vi "RDG822 User.vi"() -> ()   [LabVIEW 2021]
panel:
  in  "MenuCont":u32=1
  in  "RemoveReq?":bool=TRUE
  in  "userID":string="0001"
  out "error out":errorcluster
  in  "E:\\Study\\НИР_Маг\\FP":path=path "E:/Study/НИР_Маг/FP"
  in  "error in":errorcluster
  in  "DutyDBL":dbl=50.0 format="%.3f"
  out "DutyStr":string="50.000 %"
  in  "Noise":bool
  in  "Pulse":bool
  in  "Ramp":bool
  in  "Square":bool
  in  "Sine":bool
  in  "Slider":bool
  in  "PhaseDBL":dbl format="%.3f"
  in  "OK":bool
  out "PhaseStr":string="5.0000"
  in  "LowL":dbl=-2.5 format="%.4f"
  in  "Offset":dbl format="%.4f"
  out "Offset-LowL":string="5.0000"
  in  "Offset/LowL":bool
  in  "HighL":dbl=1.0 format="%.4f"
  in  "Ampl":dbl=5.0 format="%.4f"
  out "Ampl-HighL":string="5.0000"
  in  "Ampl/HighL":bool
  in  "Freq":dbl=1.0 format="%#_18g"
  in  "Period":dbl=1.0 format="%_8g"
  out "Freq-Period":string="1,000000000"
  in  "Freq/Period":bool
  in  "Left":bool
  in  "Right":bool
  in  "Out2":bool
  in  "Out1":bool
  out "Screen":picture
  in  "Menu":bool
  in  "Home":bool
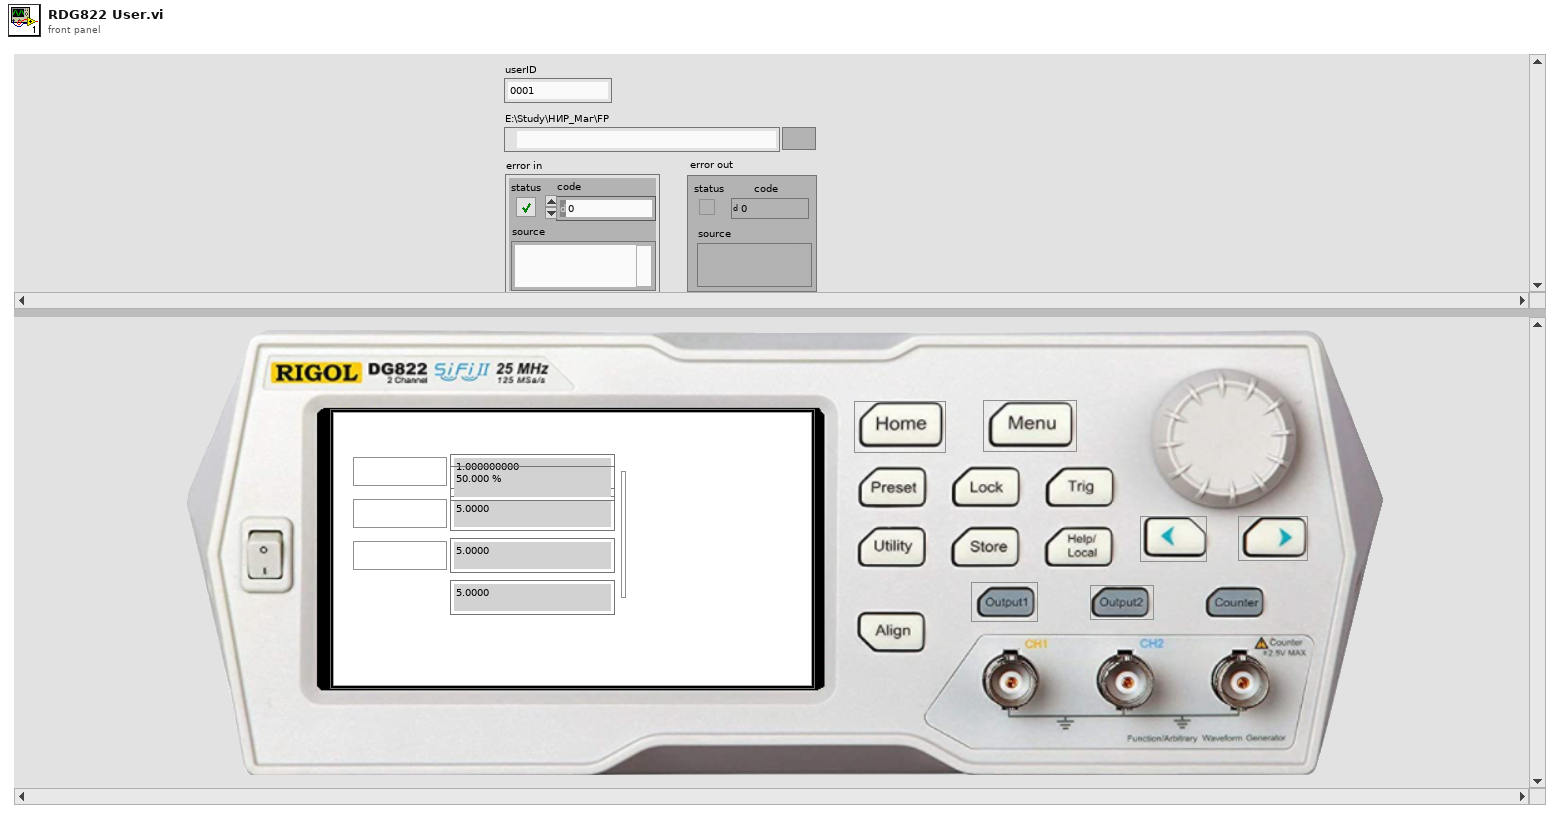
[diagram p1: front panel]
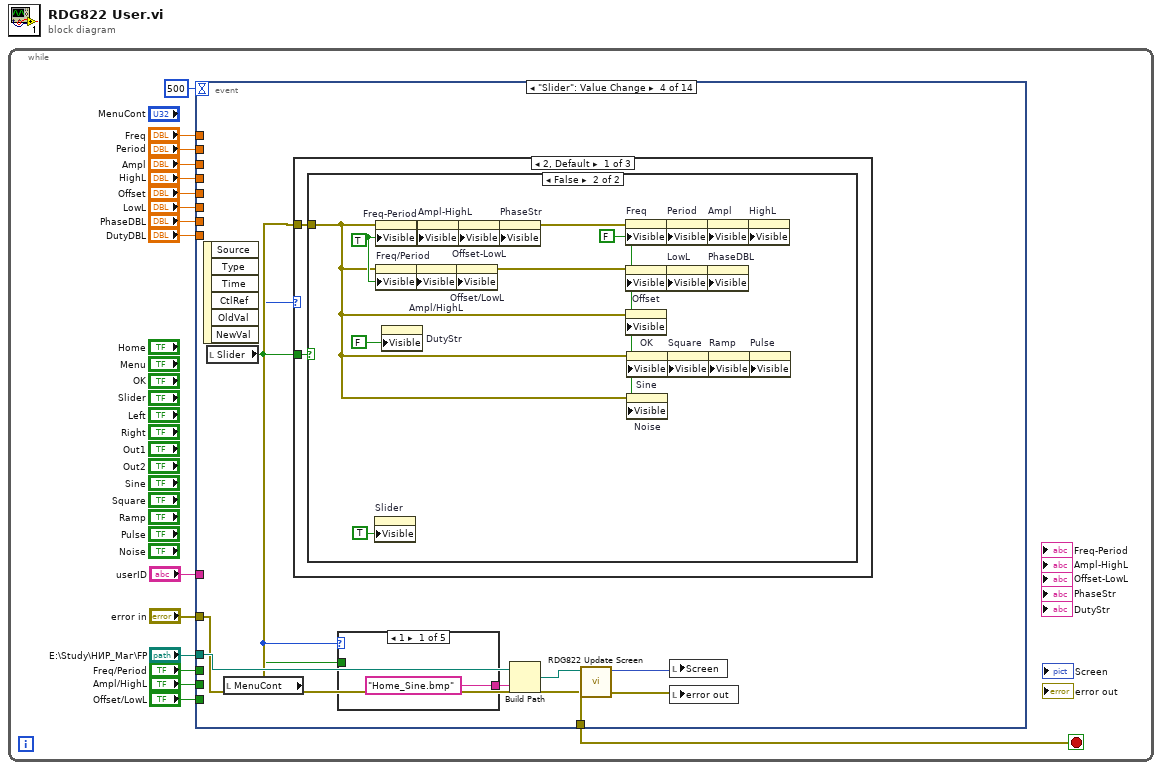
[diagram p0: block diagram]
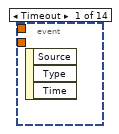
[diagram p2: hidden frame]
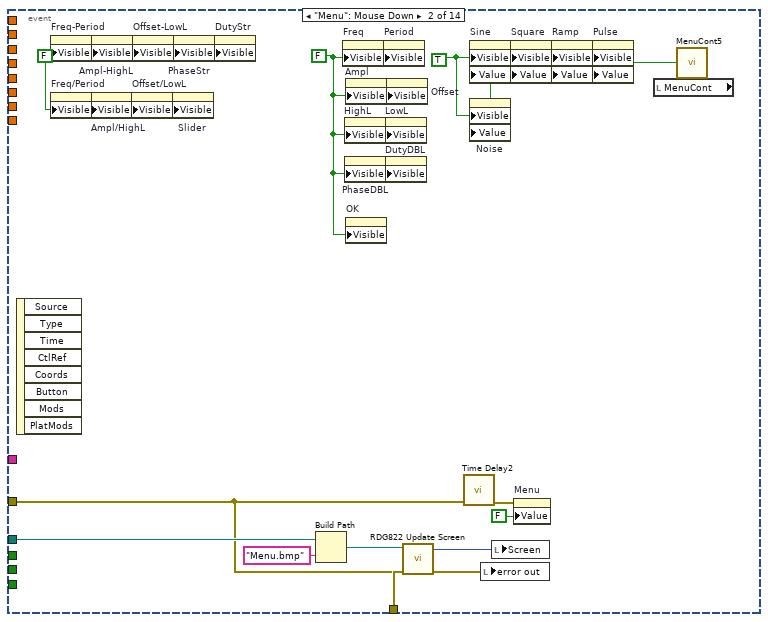
[diagram p3: hidden frame]
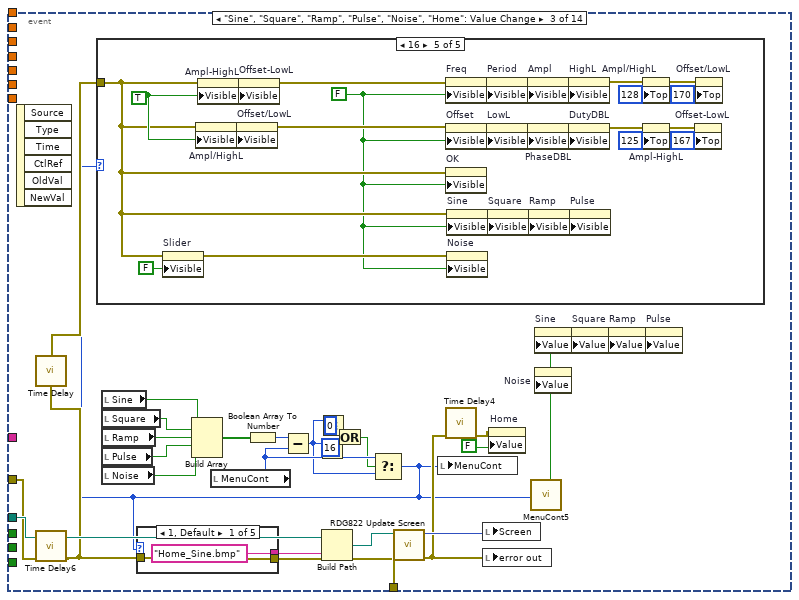
[diagram p4: hidden frame]
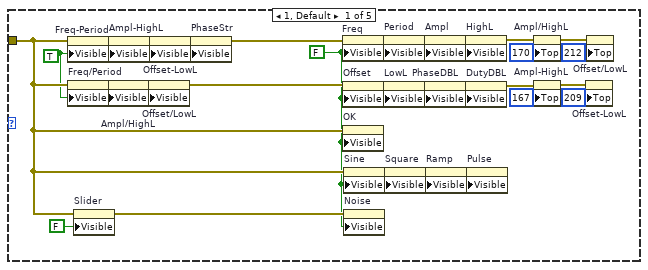
[diagram p5: hidden frame]
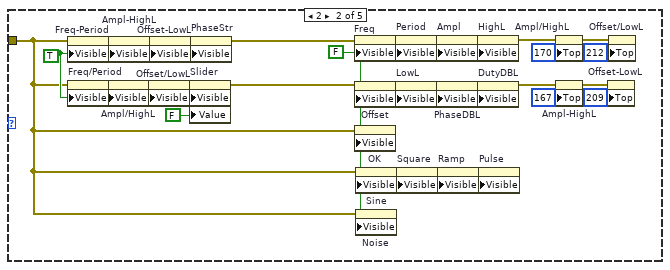
[diagram p6: hidden frame]
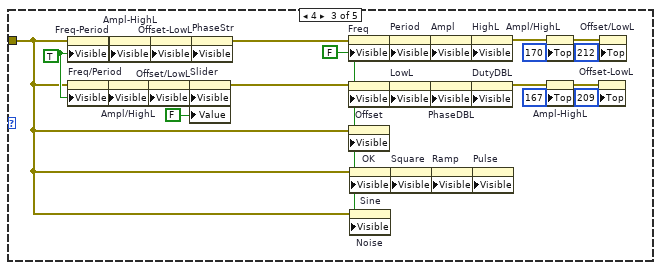
[diagram p7: hidden frame]
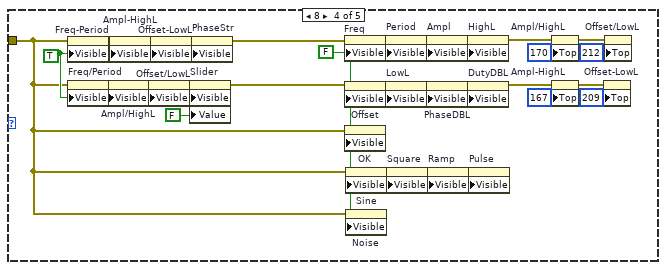
[diagram p8: hidden frame]
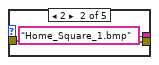
[diagram p9: hidden frame]
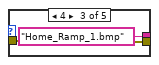
[diagram p10: hidden frame]
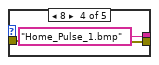
[diagram p11: hidden frame]
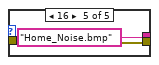
[diagram p12: hidden frame]
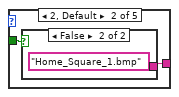
[diagram p13: hidden frame]
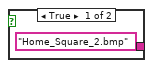
[diagram p14: hidden frame]
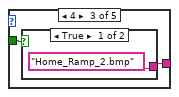
[diagram p15: hidden frame]
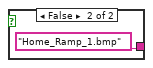
[diagram p16: hidden frame]
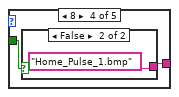
[diagram p17: hidden frame]
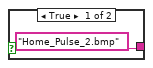
[diagram p18: hidden frame]
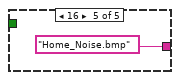
[diagram p19: hidden frame]
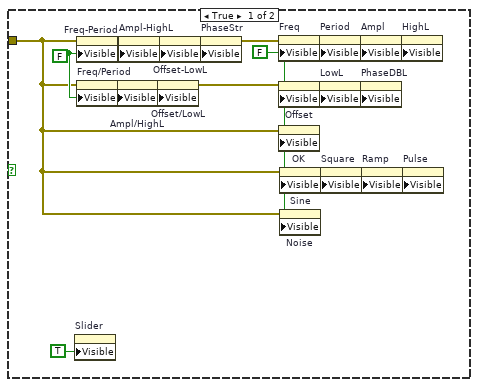
[diagram p20: hidden frame]
diagram:
  n1 = while {
    stop <- w16 stop-if-true
    n2 = event shown="[3] \"Slider\": Value Change" {
      selector: _ -> [_ _ _ _ _ _ _ _ _ _ _ _ _ _]
      dyn-events: _ -> [_ _ _ _ _ _ _ _ _ _ _ _ _ _]
      timeout: 500 -> [_ _ _ _ _ _ _ _ _ _ _ _ _ _]
      tunnel: [_ w39 w64 w229 w375 w518 w552 w587 w622 w645 _ _ w705 _] -> w16
      tunnel: "error in" -> [_ w37 w52 w228 w383 _ _ _ _ _ _ _ w723 _]
      tunnel: "E:\\Study\\НИР_Маг\\FP" -> [_ w40 w68 w230 w387 w535 w570 w605 w629 w652 _ _ w711 _]
      tunnel: "Freq/Period" -> [_ _ _ _ w390 w533 _ _ _ _ _ _ w740 _]
      tunnel: "Ampl/HighL" -> [_ _ _ _ w389 _ w565 _ _ _ _ _ w741 _]
      tunnel: "Freq" -> [_ _ _ _ _ _ _ _ _ _ _ _ w739 _]
      tunnel: "Ampl" -> [_ _ _ _ _ _ _ _ _ _ _ _ w737 _]
      tunnel: "Period" -> [_ _ _ _ _ _ _ _ _ _ _ _ w738 _]
      tunnel: "HighL" -> [_ _ _ _ _ _ _ _ _ _ _ _ w734 _]
      tunnel: "Offset/LowL" -> [_ _ _ _ w388 _ _ w593 _ _ _ _ w736 _]
      tunnel: "Offset" -> [_ _ _ _ _ _ _ _ _ _ _ _ w700 _]
      tunnel: "LowL" -> [_ _ _ _ _ _ _ _ _ _ _ _ w735 _]
      tunnel: "PhaseDBL" -> [_ _ _ _ _ _ _ _ _ _ _ _ w728 _]
      tunnel: "userID" -> [_ _ _ _ _ _ _ _ _ _ _ _ w722 _]
      tunnel: "DutyDBL" -> [_ _ _ _ _ _ _ _ _ _ _ _ w697 _]
      event Timeout {
        n3 = event-data() -> ()  [unwired: 1 in, 3 out]
      }
      event "Menu": Mouse Down {
        w25 = TRUE ("Visible")
        w18 = FALSE ("Visible")
        w17 = FALSE ("Visible")
        n4 = event-data() -> ()  [unwired: 1 in, 8 out]
        n5 = property on="Freq-Period" class="Str"("Visible"=w18) -> (error out=w36:errorcluster)  [unwired: 2 in, 1 out]
        n6 = property on="Freq/Period" class="Bool (strict)"("Visible"=w18) -> (error out=w33:errorcluster)  [unwired: 2 in, 1 out]
        n7 = property on="Ampl/HighL" class="Bool (strict)"(error in=w33, "Visible"=w18) -> (error out=w32:errorcluster)  [unwired: 1 in, 1 out]
        n8 = property on="Ampl-HighL" class="Str"(error in=w36, "Visible"=w18) -> (error out=w35:errorcluster)  [unwired: 1 in, 1 out]
        n9 = property on="Offset/LowL" class="Bool (strict)"(error in=w32, "Visible"=w18) -> (error out=w29:errorcluster)  [unwired: 1 in, 1 out]
        n10 = property on="Offset-LowL" class="Str"(error in=w35, "Visible"=w18) -> (error out=w34:errorcluster)  [unwired: 1 in, 1 out]
        n11 = property on="Slider" class="Bool (strict)"(error in=w29, "Visible"=w18) -> ()  [unwired: 1 in, 2 out]
        n12 = property on="PhaseStr" class="Str"(error in=w34, "Visible"=w18) -> ()  [unwired: 1 in, 2 out]
        n13 = property on="DutyStr" class="Str"("Visible"=w18) -> ()  [unwired: 2 in, 2 out]
        n14 = Build Path(base path=w40, name or relative path="Menu.bmp") -> (appended path=w41:path)
        n15 = property on="Freq" class="DigNum (strict)"("Visible"=w17) -> (error out=w31:errorcluster)  [unwired: 2 in, 1 out]
        n16 = property on="HighL" class="DigNum (strict)"("Visible"=w17) -> ()  [unwired: 2 in, 2 out]
        n17 = property on="PhaseDBL" class="DigNum (strict)"("Visible"=w17) -> ()  [unwired: 2 in, 2 out]
        n18 = property on="Ampl" class="DigNum (strict)"("Visible"=w17) -> (error out=w30:errorcluster)  [unwired: 2 in, 1 out]
        n19 = property on="OK" class="Bool (strict)"("Visible"=w17) -> ()  [unwired: 2 in, 2 out]
        n20 = property on="Period" class="DigNum (strict)"(error in=w31, "Visible"=w17) -> ()  [unwired: 1 in, 2 out]
        n21 = property on="LowL" class="DigNum (strict)"("Visible"=w17) -> ()  [unwired: 2 in, 2 out]
        n22 = property on="DutyDBL" class="DigNum (strict)"("Visible"=w17) -> ()  [unwired: 2 in, 2 out]
        n23 = property on="Offset" class="DigNum (strict)"(error in=w30, "Visible"=w17) -> ()  [unwired: 1 in, 2 out]
        n24 = call "RDG822 Update Screen.vi"("error in"=w37, "Path to file"=w41) -> ("error out"=w39:errorcluster, "Screen"=w38:picture)  [unwired: 8 in]
        n25 = call "Time Delay2"("error in (no error)"=w37) -> ("error out"=w44:errorcluster)  [unwired: 10 in]
        n26 = local write "error out"(w39) -> ()
        n27 = local write "Screen"(w38) -> ()
        n28 = property on="Menu" class="Bool (strict)"(error in=w44, "Value"=FALSE ("Visible")) -> ()  [unwired: 1 in, 2 out]
        n29 = local read "MenuCont"() -> (w24:u32)
        n30 = call "MenuCont5.vi"("MenuID"=w24) -> ("Sine"=w23:bool, "Square"=w22:bool, "Ramp"=w21:bool, "Pulse"=w20:bool, "Noise"=w19:bool)  [unwired: 10 in]
        n31 = property on="Sine" class="Bool (strict)"("Visible"=w25, "Value"=w23) -> (error out=w28:errorcluster)  [unwired: 2 in, 1 out]
        n32 = property on="Noise" class="Bool (strict)"("Visible"=w25, "Value"=w19) -> ()  [unwired: 2 in, 2 out]
        n33 = property on="Square" class="Bool (strict)"(error in=w28, "Visible"=w25, "Value"=w22) -> (error out=w27:errorcluster)  [unwired: 1 in, 1 out]
        n34 = property on="Ramp" class="Bool (strict)"(error in=w27, "Visible"=w25, "Value"=w21) -> (error out=w26:errorcluster)  [unwired: 1 in, 1 out]
        n35 = property on="Pulse" class="Bool (strict)"(error in=w26, "Visible"=w25, "Value"=w20) -> ()  [unwired: 1 in, 2 out]
      }
      event "Sine", "Square", "Ramp", "Pulse", "Noise", "Home": Value Change {
        n36 = event-data() -> ()  [unwired: 1 in, 6 out]
        n37 = call "Time Delay6"("error in (no error)"=w52) -> ("error out"=w49:errorcluster)  [unwired: 10 in]
        n38 = call "Time Delay"("error in (no error)"=w49) -> ("error out"=w50:errorcluster)  [unwired: 10 in]
        n39 = local read "Sine"() -> (w73:bool)
        n40 = local read "Square"() -> (w74:bool)
        n41 = local read "Ramp"() -> (w75:bool)
        n42 = local read "Pulse"() -> (w72:bool)
        n43 = local read "Noise"() -> (w71:bool)
        n44 = Build Array(w73, w74, w75, w72, w71) -> (w76:bool[])
        n45 = local read "MenuCont"() -> (w48:u32)
        n46 = Boolean Array To Number(Boolean array=w76) -> (number=w70:u32)
        n47 = Subtract(x=w70, y=w48) -> (x-y=w47:u32)
        n48 = Greater?(x=w47, y=u32 16) -> (0:w54:bool)
        n49 = Less Or Equal?(x=w47, y=u32 0) -> (x <= y?=w55:bool)
        n50 = Or(x=w55, y=w54) -> (x .or. y?=w46:bool)
        n51 = Select(t=w48, s=w46, f=w47) -> (s? t:f=w45:u32)
        n52 = case shown="16" w45 {
          tunnel: w50 -> [w90 w117 w145 w173 w200]
          frame 1, Default {
            w79 = TRUE ("Visible")
            w80 = FALSE ("Visible")
            n53 = property on="Freq-Period" class="Str"(error in=w90, "Visible"=w79) -> (error out=w106:errorcluster)  [unwired: 1 in, 1 out]
            n54 = property on="Freq/Period" class="Bool (strict)"(error in=w90, "Visible"=w79) -> (error out=w103:errorcluster)  [unwired: 1 in, 1 out]
            n55 = property on="Slider" class="Bool (strict)"(error in=w90, "Visible"=FALSE) -> (error out=w91:errorcluster)  [unwired: 1 in, 1 out]
            n56 = property on="Ampl/HighL" class="Bool (strict)"(error in=w103, "Visible"=w79) -> (error out=w102:errorcluster)  [unwired: 1 in, 1 out]
            n57 = property on="Ampl-HighL" class="Str"(error in=w106, "Visible"=w79) -> (error out=w105:errorcluster)  [unwired: 1 in, 1 out]
            n58 = property on="Offset/LowL" class="Bool (strict)"(error in=w102, "Visible"=w79) -> (error out=w92:errorcluster)  [unwired: 1 in, 1 out]
            n59 = property on="Offset-LowL" class="Str"(error in=w105, "Visible"=w79) -> (error out=w104:errorcluster)  [unwired: 1 in, 1 out]
            n60 = property on="PhaseStr" class="Str"(error in=w104, "Visible"=w79) -> (error out=w97:errorcluster)  [unwired: 1 in, 1 out]
            n61 = property on="Freq" class="DigNum (strict)"(error in=w97, "Visible"=w80) -> (error out=w96:errorcluster)  [unwired: 1 in, 1 out]
            n62 = property on="Offset" class="DigNum (strict)"(error in=w92, "Visible"=w80) -> (error out=w93:errorcluster)  [unwired: 1 in, 1 out]
            n63 = property on="OK" class="Bool (strict)"(error in=w90, "Visible"=w80) -> ()  [unwired: 1 in, 2 out]
            n64 = property on="Sine" class="Bool (strict)"(error in=w90, "Visible"=w80) -> (error out=w100:errorcluster)  [unwired: 1 in, 1 out]
            n65 = property on="Noise" class="Bool (strict)"(error in=w91, "Visible"=w80) -> ()  [unwired: 1 in, 2 out]
            n66 = property on="Period" class="DigNum (strict)"(error in=w96, "Visible"=w80) -> (error out=w95:errorcluster)  [unwired: 1 in, 1 out]
            n67 = property on="LowL" class="DigNum (strict)"(error in=w93, "Visible"=w80) -> (error out=w94:errorcluster)  [unwired: 1 in, 1 out]
            n68 = property on="Square" class="Bool (strict)"(error in=w100, "Visible"=w80) -> (error out=w99:errorcluster)  [unwired: 1 in, 1 out]
            n69 = property on="Ampl" class="DigNum (strict)"(error in=w95, "Visible"=w80) -> (error out=w101:errorcluster)  [unwired: 1 in, 1 out]
            n70 = property on="PhaseDBL" class="DigNum (strict)"(error in=w94, "Visible"=w80) -> (error out=w81:errorcluster)  [unwired: 1 in, 1 out]
            n71 = property on="Ramp" class="Bool (strict)"(error in=w99, "Visible"=w80) -> (error out=w98:errorcluster)  [unwired: 1 in, 1 out]
            n72 = property on="HighL" class="DigNum (strict)"(error in=w101, "Visible"=w80) -> (error out=w87:errorcluster)  [unwired: 1 in, 1 out]
            n73 = property on="DutyDBL" class="DigNum (strict)"("Visible"=w80) -> ()  [unwired: 2 in, 2 out]
            n74 = property on="Pulse" class="Bool (strict)"(error in=w98, "Visible"=w80) -> ()  [unwired: 1 in, 2 out]
            n75 = property on="Ampl/HighL" class="Bool (strict)"(error in=w87, "Top"=170 ("Position:Top")) -> (error out=w85:errorcluster)  [unwired: 1 in, 1 out]
            n76 = property on="Ampl-HighL" class="Str"(error in=w81, "Top"=167 ("Position:Top")) -> (error out=w82:errorcluster)  [unwired: 1 in, 1 out]
            n77 = property on="Offset-LowL" class="Str"(error in=w82, "Top"=209 ("Position:Top")) -> ()  [unwired: 1 in, 2 out]
            n78 = property on="Offset/LowL" class="Bool (strict)"(error in=w85, "Top"=212 ("Position:Top")) -> ()  [unwired: 1 in, 2 out]
          }
          frame 2 {
            w127 = TRUE ("Visible")
            w107 = FALSE ("Visible")
            n79 = property on="Freq-Period" class="Str"(error in=w117, "Visible"=w127) -> (error out=w134:errorcluster)  [unwired: 1 in, 1 out]
            n80 = property on="Freq/Period" class="Bool (strict)"(error in=w117, "Visible"=w127) -> (error out=w131:errorcluster)  [unwired: 1 in, 1 out]
            n81 = property on="Ampl/HighL" class="Bool (strict)"(error in=w131, "Visible"=w127) -> (error out=w130:errorcluster)  [unwired: 1 in, 1 out]
            n82 = property on="Ampl-HighL" class="Str"(error in=w134, "Visible"=w127) -> (error out=w133:errorcluster)  [unwired: 1 in, 1 out]
            n83 = property on="Offset/LowL" class="Bool (strict)"(error in=w130, "Visible"=w127) -> (error out=w128:errorcluster)  [unwired: 1 in, 1 out]
            n84 = property on="Offset-LowL" class="Str"(error in=w133, "Visible"=w127) -> (error out=w132:errorcluster)  [unwired: 1 in, 1 out]
            n85 = property on="Slider" class="Bool (strict)"(error in=w128, "Visible"=w127, "Value"=FALSE ("Slider")) -> (error out=w122:errorcluster)  [unwired: 1 in, 1 out]
            n86 = property on="PhaseStr" class="Str"(error in=w132, "Visible"=w127) -> (error out=w123:errorcluster)  [unwired: 1 in, 1 out]
            n87 = property on="Freq" class="DigNum (strict)"(error in=w123, "Visible"=w107) -> (error out=w121:errorcluster)  [unwired: 1 in, 1 out]
            n88 = property on="Offset" class="DigNum (strict)"(error in=w122, "Visible"=w107) -> (error out=w118:errorcluster)  [unwired: 1 in, 1 out]
            n89 = property on="OK" class="Bool (strict)"(error in=w117, "Visible"=w107) -> ()  [unwired: 1 in, 2 out]
            n90 = property on="Sine" class="Bool (strict)"(error in=w117, "Visible"=w107) -> (error out=w126:errorcluster)  [unwired: 1 in, 1 out]
            n91 = property on="Noise" class="Bool (strict)"(error in=w117, "Visible"=w107) -> ()  [unwired: 1 in, 2 out]
            n92 = property on="Period" class="DigNum (strict)"(error in=w121, "Visible"=w107) -> (error out=w120:errorcluster)  [unwired: 1 in, 1 out]
            n93 = property on="LowL" class="DigNum (strict)"(error in=w118, "Visible"=w107) -> (error out=w119:errorcluster)  [unwired: 1 in, 1 out]
            n94 = property on="Square" class="Bool (strict)"(error in=w126, "Visible"=w107) -> (error out=w125:errorcluster)  [unwired: 1 in, 1 out]
            n95 = property on="Ampl" class="DigNum (strict)"(error in=w120, "Visible"=w107) -> (error out=w129:errorcluster)  [unwired: 1 in, 1 out]
            n96 = property on="PhaseDBL" class="DigNum (strict)"(error in=w119, "Visible"=w107) -> (error out=w109:errorcluster)  [unwired: 1 in, 1 out]
            n97 = property on="Ramp" class="Bool (strict)"(error in=w125, "Visible"=w107) -> (error out=w124:errorcluster)  [unwired: 1 in, 1 out]
            n98 = property on="HighL" class="DigNum (strict)"(error in=w129, "Visible"=w107) -> (error out=w108:errorcluster)  [unwired: 1 in, 1 out]
            n99 = property on="DutyDBL" class="DigNum (strict)"("Visible"=w107) -> ()  [unwired: 2 in, 2 out]
            n100 = property on="Pulse" class="Bool (strict)"(error in=w124, "Visible"=w107) -> ()  [unwired: 1 in, 2 out]
            n101 = property on="Ampl/HighL" class="Bool (strict)"(error in=w108, "Top"=170 ("Position:Top")) -> (error out=w113:errorcluster)  [unwired: 1 in, 1 out]
            n102 = property on="Ampl-HighL" class="Str"(error in=w109, "Top"=167 ("Position:Top")) -> (error out=w110:errorcluster)  [unwired: 1 in, 1 out]
            n103 = property on="Offset-LowL" class="Str"(error in=w110, "Top"=209 ("Position:Top")) -> ()  [unwired: 1 in, 2 out]
            n104 = property on="Offset/LowL" class="Bool (strict)"(error in=w113, "Top"=212 ("Position:Top")) -> ()  [unwired: 1 in, 2 out]
          }
          frame 4 {
            w155 = TRUE ("Visible")
            w135 = FALSE ("Visible")
            n105 = property on="Freq-Period" class="Str"(error in=w145, "Visible"=w155) -> (error out=w162:errorcluster)  [unwired: 1 in, 1 out]
            n106 = property on="Freq/Period" class="Bool (strict)"(error in=w145, "Visible"=w155) -> (error out=w159:errorcluster)  [unwired: 1 in, 1 out]
            n107 = property on="Ampl/HighL" class="Bool (strict)"(error in=w159, "Visible"=w155) -> (error out=w158:errorcluster)  [unwired: 1 in, 1 out]
            n108 = property on="Ampl-HighL" class="Str"(error in=w162, "Visible"=w155) -> (error out=w161:errorcluster)  [unwired: 1 in, 1 out]
            n109 = property on="Offset/LowL" class="Bool (strict)"(error in=w158, "Visible"=w155) -> (error out=w156:errorcluster)  [unwired: 1 in, 1 out]
            n110 = property on="Offset-LowL" class="Str"(error in=w161, "Visible"=w155) -> (error out=w160:errorcluster)  [unwired: 1 in, 1 out]
            n111 = property on="Slider" class="Bool (strict)"(error in=w156, "Visible"=w155, "Value"=FALSE ("Slider")) -> (error out=w150:errorcluster)  [unwired: 1 in, 1 out]
            n112 = property on="PhaseStr" class="Str"(error in=w160, "Visible"=w155) -> (error out=w151:errorcluster)  [unwired: 1 in, 1 out]
            n113 = property on="Freq" class="DigNum (strict)"(error in=w151, "Visible"=w135) -> (error out=w149:errorcluster)  [unwired: 1 in, 1 out]
            n114 = property on="Offset" class="DigNum (strict)"(error in=w150, "Visible"=w135) -> (error out=w146:errorcluster)  [unwired: 1 in, 1 out]
            n115 = property on="OK" class="Bool (strict)"(error in=w145, "Visible"=w135) -> ()  [unwired: 1 in, 2 out]
            n116 = property on="Sine" class="Bool (strict)"(error in=w145, "Visible"=w135) -> (error out=w154:errorcluster)  [unwired: 1 in, 1 out]
            n117 = property on="Noise" class="Bool (strict)"(error in=w145, "Visible"=w135) -> ()  [unwired: 1 in, 2 out]
            n118 = property on="Period" class="DigNum (strict)"(error in=w149, "Visible"=w135) -> (error out=w148:errorcluster)  [unwired: 1 in, 1 out]
            n119 = property on="LowL" class="DigNum (strict)"(error in=w146, "Visible"=w135) -> (error out=w147:errorcluster)  [unwired: 1 in, 1 out]
            n120 = property on="Square" class="Bool (strict)"(error in=w154, "Visible"=w135) -> (error out=w153:errorcluster)  [unwired: 1 in, 1 out]
            n121 = property on="Ampl" class="DigNum (strict)"(error in=w148, "Visible"=w135) -> (error out=w157:errorcluster)  [unwired: 1 in, 1 out]
            n122 = property on="PhaseDBL" class="DigNum (strict)"(error in=w147, "Visible"=w135) -> (error out=w136:errorcluster)  [unwired: 1 in, 1 out]
            n123 = property on="Ramp" class="Bool (strict)"(error in=w153, "Visible"=w135) -> (error out=w152:errorcluster)  [unwired: 1 in, 1 out]
            n124 = property on="HighL" class="DigNum (strict)"(error in=w157, "Visible"=w135) -> (error out=w137:errorcluster)  [unwired: 1 in, 1 out]
            n125 = property on="DutyDBL" class="DigNum (strict)"("Visible"=w135) -> ()  [unwired: 2 in, 2 out]
            n126 = property on="Pulse" class="Bool (strict)"(error in=w152, "Visible"=w135) -> ()  [unwired: 1 in, 2 out]
            n127 = property on="Ampl/HighL" class="Bool (strict)"(error in=w137, "Top"=170 ("Position:Top")) -> (error out=w141:errorcluster)  [unwired: 1 in, 1 out]
            n128 = property on="Ampl-HighL" class="Str"(error in=w136, "Top"=167 ("Position:Top")) -> (error out=w138:errorcluster)  [unwired: 1 in, 1 out]
            n129 = property on="Offset-LowL" class="Str"(error in=w138, "Top"=209 ("Position:Top")) -> ()  [unwired: 1 in, 2 out]
            n130 = property on="Offset/LowL" class="Bool (strict)"(error in=w141, "Top"=212 ("Position:Top")) -> ()  [unwired: 1 in, 2 out]
          }
          frame 8 {
            w183 = TRUE ("Visible")
            w163 = FALSE ("Visible")
            n131 = property on="Freq-Period" class="Str"(error in=w173, "Visible"=w183) -> (error out=w190:errorcluster)  [unwired: 1 in, 1 out]
            n132 = property on="Freq/Period" class="Bool (strict)"(error in=w173, "Visible"=w183) -> (error out=w187:errorcluster)  [unwired: 1 in, 1 out]
            n133 = property on="Ampl/HighL" class="Bool (strict)"(error in=w187, "Visible"=w183) -> (error out=w186:errorcluster)  [unwired: 1 in, 1 out]
            n134 = property on="Ampl-HighL" class="Str"(error in=w190, "Visible"=w183) -> (error out=w189:errorcluster)  [unwired: 1 in, 1 out]
            n135 = property on="Offset/LowL" class="Bool (strict)"(error in=w186, "Visible"=w183) -> (error out=w184:errorcluster)  [unwired: 1 in, 1 out]
            n136 = property on="Offset-LowL" class="Str"(error in=w189, "Visible"=w183) -> (error out=w188:errorcluster)  [unwired: 1 in, 1 out]
            n137 = property on="Slider" class="Bool (strict)"(error in=w184, "Visible"=w183, "Value"=FALSE ("Slider")) -> (error out=w178:errorcluster)  [unwired: 1 in, 1 out]
            n138 = property on="PhaseStr" class="Str"(error in=w188, "Visible"=w183) -> (error out=w179:errorcluster)  [unwired: 1 in, 1 out]
            n139 = property on="Freq" class="DigNum (strict)"(error in=w179, "Visible"=w163) -> (error out=w177:errorcluster)  [unwired: 1 in, 1 out]
            n140 = property on="Offset" class="DigNum (strict)"(error in=w178, "Visible"=w163) -> (error out=w174:errorcluster)  [unwired: 1 in, 1 out]
            n141 = property on="OK" class="Bool (strict)"(error in=w173, "Visible"=w163) -> ()  [unwired: 1 in, 2 out]
            n142 = property on="Sine" class="Bool (strict)"(error in=w173, "Visible"=w163) -> (error out=w182:errorcluster)  [unwired: 1 in, 1 out]
            n143 = property on="Noise" class="Bool (strict)"(error in=w173, "Visible"=w163) -> ()  [unwired: 1 in, 2 out]
            n144 = property on="Period" class="DigNum (strict)"(error in=w177, "Visible"=w163) -> (error out=w176:errorcluster)  [unwired: 1 in, 1 out]
            n145 = property on="LowL" class="DigNum (strict)"(error in=w174, "Visible"=w163) -> (error out=w175:errorcluster)  [unwired: 1 in, 1 out]
            n146 = property on="Square" class="Bool (strict)"(error in=w182, "Visible"=w163) -> (error out=w181:errorcluster)  [unwired: 1 in, 1 out]
            n147 = property on="Ampl" class="DigNum (strict)"(error in=w176, "Visible"=w163) -> (error out=w185:errorcluster)  [unwired: 1 in, 1 out]
            n148 = property on="PhaseDBL" class="DigNum (strict)"(error in=w175, "Visible"=w163) -> (error out=w164:errorcluster)  [unwired: 1 in, 1 out]
            n149 = property on="Ramp" class="Bool (strict)"(error in=w181, "Visible"=w163) -> (error out=w180:errorcluster)  [unwired: 1 in, 1 out]
            n150 = property on="HighL" class="DigNum (strict)"(error in=w185, "Visible"=w163) -> (error out=w165:errorcluster)  [unwired: 1 in, 1 out]
            n151 = property on="DutyDBL" class="DigNum (strict)"("Visible"=w163) -> ()  [unwired: 2 in, 2 out]
            n152 = property on="Pulse" class="Bool (strict)"(error in=w180, "Visible"=w163) -> ()  [unwired: 1 in, 2 out]
            n153 = property on="Ampl/HighL" class="Bool (strict)"(error in=w165, "Top"=170 ("Position:Top")) -> (error out=w169:errorcluster)  [unwired: 1 in, 1 out]
            n154 = property on="Ampl-HighL" class="Str"(error in=w164, "Top"=167 ("Position:Top")) -> (error out=w166:errorcluster)  [unwired: 1 in, 1 out]
            n155 = property on="Offset-LowL" class="Str"(error in=w166, "Top"=209 ("Position:Top")) -> ()  [unwired: 1 in, 2 out]
            n156 = property on="Offset/LowL" class="Bool (strict)"(error in=w169, "Top"=212 ("Position:Top")) -> ()  [unwired: 1 in, 2 out]
          }
          frame 16 {
            w211 = TRUE ("Visible")
            w191 = FALSE ("Visible")
            n157 = property on="Slider" class="Bool (strict)"(error in=w200, "Visible"=FALSE) -> ()  [unwired: 1 in, 2 out]
            n158 = property on="Ampl/HighL" class="Bool (strict)"(error in=w200, "Visible"=w211) -> (error out=w213:errorcluster)  [unwired: 1 in, 1 out]
            n159 = property on="Ampl-HighL" class="Str"(error in=w200, "Visible"=w211) -> (error out=w214:errorcluster)  [unwired: 1 in, 1 out]
            n160 = property on="Offset/LowL" class="Bool (strict)"(error in=w213, "Visible"=w211) -> (error out=w203:errorcluster)  [unwired: 1 in, 1 out]
            n161 = property on="Offset-LowL" class="Str"(error in=w214, "Visible"=w211) -> (error out=w201:errorcluster)  [unwired: 1 in, 1 out]
            n162 = property on="Freq" class="DigNum (strict)"(error in=w201, "Visible"=w191) -> (error out=w207:errorcluster)  [unwired: 1 in, 1 out]
            n163 = property on="Offset" class="DigNum (strict)"(error in=w203, "Visible"=w191) -> (error out=w204:errorcluster)  [unwired: 1 in, 1 out]
            n164 = property on="OK" class="Bool (strict)"(error in=w200, "Visible"=w191) -> ()  [unwired: 1 in, 2 out]
            n165 = property on="Sine" class="Bool (strict)"(error in=w200, "Visible"=w191) -> (error out=w210:errorcluster)  [unwired: 1 in, 1 out]
            n166 = property on="Noise" class="Bool (strict)"(error in=w200, "Visible"=w191) -> ()  [unwired: 1 in, 2 out]
            n167 = property on="Period" class="DigNum (strict)"(error in=w207, "Visible"=w191) -> (error out=w206:errorcluster)  [unwired: 1 in, 1 out]
            n168 = property on="LowL" class="DigNum (strict)"(error in=w204, "Visible"=w191) -> (error out=w205:errorcluster)  [unwired: 1 in, 1 out]
            n169 = property on="Square" class="Bool (strict)"(error in=w210, "Visible"=w191) -> (error out=w209:errorcluster)  [unwired: 1 in, 1 out]
            n170 = property on="Ampl" class="DigNum (strict)"(error in=w206, "Visible"=w191) -> (error out=w212:errorcluster)  [unwired: 1 in, 1 out]
            n171 = property on="PhaseDBL" class="DigNum (strict)"(error in=w205, "Visible"=w191) -> (error out=w192:errorcluster)  [unwired: 1 in, 1 out]
            n172 = property on="Ramp" class="Bool (strict)"(error in=w209, "Visible"=w191) -> (error out=w208:errorcluster)  [unwired: 1 in, 1 out]
            n173 = property on="HighL" class="DigNum (strict)"(error in=w212, "Visible"=w191) -> (error out=w193:errorcluster)  [unwired: 1 in, 1 out]
            n174 = property on="DutyDBL" class="DigNum (strict)"("Visible"=w191) -> ()  [unwired: 2 in, 2 out]
            n175 = property on="Pulse" class="Bool (strict)"(error in=w208, "Visible"=w191) -> ()  [unwired: 1 in, 2 out]
            n176 = property on="Ampl/HighL" class="Bool (strict)"(error in=w193, "Top"=128 ("Position:Top")) -> (error out=w197:errorcluster)  [unwired: 1 in, 1 out]
            n177 = property on="Ampl-HighL" class="Str"(error in=w192, "Top"=125 ("Position:Top")) -> (error out=w194:errorcluster)  [unwired: 1 in, 1 out]
            n178 = property on="Offset-LowL" class="Str"(error in=w194, "Top"=167 ("Position:Top")) -> ()  [unwired: 1 in, 2 out]
            n179 = property on="Offset/LowL" class="Bool (strict)"(error in=w197, "Top"=170 ("Position:Top")) -> ()  [unwired: 1 in, 2 out]
          }
        }
        n180 = case shown="1, Default" w45 {
          tunnel: ["Home_Sine.bmp" "Home_Square_1.bmp" "Home_Ramp_1.bmp" "Home_Pulse_1.bmp" "Home_Noise.bmp"] -> w69
          tunnel: w49 -> [w215 w217 w219 w221 w223]
          tunnel: [w215 w217 w219 w221 w223] -> w51
          frame 1, Default {
          }
          frame 2 {
          }
          frame 4 {
          }
          frame 8 {
          }
          frame 16 {
          }
        }
        n181 = Build Path(base path=w68, name or relative path=w69) -> (appended path=w78:path)
        n182 = call "RDG822 Update Screen.vi"("error in"=w51, "Path to file"=w78) -> ("error out"=w64:errorcluster, "Screen"=w77:picture)  [unwired: 8 in]
        n183 = local write "MenuCont"(w45) -> ()
        n184 = call "Time Delay4"("error in (no error)"=w64) -> ("error out"=w66:errorcluster)  [unwired: 10 in]
        n185 = local write "Screen"(w77) -> ()
        n186 = local write "error out"(w64) -> ()
        n187 = property on="Home" class="Bool (strict)"(error in=w66, "Value"=FALSE ("Home")) -> ()  [unwired: 1 in, 2 out]
        n188 = call "MenuCont5.vi"("MenuID"=w45) -> ("Sine"=w60:bool, "Square"=w59:bool, "Ramp"=w58:bool, "Pulse"=w57:bool, "Noise"=w56:bool)  [unwired: 10 in]
        n189 = property on="Sine" class="Bool (strict)"("Value"=w60) -> (error out=w63:errorcluster)  [unwired: 2 in, 1 out]
        n190 = property on="Noise" class="Bool (strict)"("Value"=w56) -> ()  [unwired: 2 in, 2 out]
        n191 = property on="Square" class="Bool (strict)"(error in=w63, "Value"=w59) -> (error out=w62:errorcluster)  [unwired: 1 in, 1 out]
        n192 = property on="Ramp" class="Bool (strict)"(error in=w62, "Value"=w58) -> (error out=w61:errorcluster)  [unwired: 1 in, 1 out]
        n193 = property on="Pulse" class="Bool (strict)"(error in=w61, "Value"=w57) -> ()  [unwired: 1 in, 2 out]
      }
      event "Slider": Value Change {
        n194 = event-data() -> ()  [unwired: 1 in, 6 out]
        n195 = local read "Slider"() -> (w226:bool)
        n196 = local read "MenuCont"() -> (w227:u32)
        n197 = case shown="2, Default" w227 {
          tunnel: w228 -> [w248 w289 w329]
          tunnel: w226 -> [w247 w288 w328]
          frame 2, Default {
            n198 = case shown="False" w247 {
              tunnel: w248 -> [w251 w271]
              frame True {
                w261 = FALSE ("Visible")
                w257 = FALSE ("Visible")
                n199 = property on="Slider" class="Bool (strict)"("Visible"=TRUE) -> ()  [unwired: 2 in, 2 out]
                n200 = property on="Freq-Period" class="Str"(error in=w251, "Visible"=w261) -> (error out=w267:errorcluster)  [unwired: 1 in, 1 out]
                n201 = property on="Freq/Period" class="Bool (strict)"(error in=w251, "Visible"=w261) -> (error out=w264:errorcluster)  [unwired: 1 in, 1 out]
                n202 = property on="Ampl/HighL" class="Bool (strict)"(error in=w264, "Visible"=w261) -> (error out=w263:errorcluster)  [unwired: 1 in, 1 out]
                n203 = property on="Ampl-HighL" class="Str"(error in=w267, "Visible"=w261) -> (error out=w266:errorcluster)  [unwired: 1 in, 1 out]
                n204 = property on="Offset/LowL" class="Bool (strict)"(error in=w263, "Visible"=w261) -> (error out=w250:errorcluster)  [unwired: 1 in, 1 out]
                n205 = property on="Offset-LowL" class="Str"(error in=w266, "Visible"=w261) -> (error out=w265:errorcluster)  [unwired: 1 in, 1 out]
                n206 = property on="PhaseStr" class="Str"(error in=w265, "Visible"=w261) -> (error out=w256:errorcluster)  [unwired: 1 in, 1 out]
                n207 = property on="Freq" class="DigNum (strict)"(error in=w256, "Visible"=w257) -> (error out=w255:errorcluster)  [unwired: 1 in, 1 out]
                n208 = property on="Offset" class="DigNum (strict)"(error in=w250, "Visible"=w257) -> (error out=w252:errorcluster)  [unwired: 1 in, 1 out]
                n209 = property on="OK" class="Bool (strict)"(error in=w251, "Visible"=w257) -> ()  [unwired: 1 in, 2 out]
                n210 = property on="Sine" class="Bool (strict)"(error in=w251, "Visible"=w257) -> (error out=w260:errorcluster)  [unwired: 1 in, 1 out]
                n211 = property on="Noise" class="Bool (strict)"(error in=w251, "Visible"=w257) -> ()  [unwired: 1 in, 2 out]
                n212 = property on="Period" class="DigNum (strict)"(error in=w255, "Visible"=w257) -> (error out=w254:errorcluster)  [unwired: 1 in, 1 out]
                n213 = property on="LowL" class="DigNum (strict)"(error in=w252, "Visible"=w257) -> (error out=w253:errorcluster)  [unwired: 1 in, 1 out]
                n214 = property on="Square" class="Bool (strict)"(error in=w260, "Visible"=w257) -> (error out=w259:errorcluster)  [unwired: 1 in, 1 out]
                n215 = property on="Ampl" class="DigNum (strict)"(error in=w254, "Visible"=w257) -> (error out=w262:errorcluster)  [unwired: 1 in, 1 out]
                n216 = property on="PhaseDBL" class="DigNum (strict)"(error in=w253, "Visible"=w257) -> ()  [unwired: 1 in, 2 out]
                n217 = property on="Ramp" class="Bool (strict)"(error in=w259, "Visible"=w257) -> (error out=w258:errorcluster)  [unwired: 1 in, 1 out]
                n218 = property on="HighL" class="DigNum (strict)"(error in=w262, "Visible"=w257) -> ()  [unwired: 1 in, 2 out]
                n219 = property on="Pulse" class="Bool (strict)"(error in=w258, "Visible"=w257) -> ()  [unwired: 1 in, 2 out]
              }
              frame False {
                w281 = TRUE ("Visible")
                w277 = FALSE ("Visible")
                n220 = property on="Slider" class="Bool (strict)"("Visible"=TRUE) -> ()  [unwired: 2 in, 2 out]
                n221 = property on="Freq-Period" class="Str"(error in=w271, "Visible"=w281) -> (error out=w287:errorcluster)  [unwired: 1 in, 1 out]
                n222 = property on="Freq/Period" class="Bool (strict)"(error in=w271, "Visible"=w281) -> (error out=w284:errorcluster)  [unwired: 1 in, 1 out]
                n223 = property on="DutyStr" class="Str"("Visible"=FALSE) -> ()  [unwired: 2 in, 2 out]
                n224 = property on="Ampl/HighL" class="Bool (strict)"(error in=w284, "Visible"=w281) -> (error out=w283:errorcluster)  [unwired: 1 in, 1 out]
                n225 = property on="Ampl-HighL" class="Str"(error in=w287, "Visible"=w281) -> (error out=w286:errorcluster)  [unwired: 1 in, 1 out]
                n226 = property on="Offset/LowL" class="Bool (strict)"(error in=w283, "Visible"=w281) -> (error out=w270:errorcluster)  [unwired: 1 in, 1 out]
                n227 = property on="Offset-LowL" class="Str"(error in=w286, "Visible"=w281) -> (error out=w285:errorcluster)  [unwired: 1 in, 1 out]
                n228 = property on="PhaseStr" class="Str"(error in=w285, "Visible"=w281) -> (error out=w276:errorcluster)  [unwired: 1 in, 1 out]
                n229 = property on="Freq" class="DigNum (strict)"(error in=w276, "Visible"=w277) -> (error out=w275:errorcluster)  [unwired: 1 in, 1 out]
                n230 = property on="Offset" class="DigNum (strict)"(error in=w270, "Visible"=w277) -> (error out=w272:errorcluster)  [unwired: 1 in, 1 out]
                n231 = property on="OK" class="Bool (strict)"(error in=w271, "Visible"=w277) -> ()  [unwired: 1 in, 2 out]
                n232 = property on="Sine" class="Bool (strict)"(error in=w271, "Visible"=w277) -> (error out=w280:errorcluster)  [unwired: 1 in, 1 out]
                n233 = property on="Noise" class="Bool (strict)"(error in=w271, "Visible"=w277) -> ()  [unwired: 1 in, 2 out]
                n234 = property on="Period" class="DigNum (strict)"(error in=w275, "Visible"=w277) -> (error out=w274:errorcluster)  [unwired: 1 in, 1 out]
                n235 = property on="LowL" class="DigNum (strict)"(error in=w272, "Visible"=w277) -> (error out=w273:errorcluster)  [unwired: 1 in, 1 out]
                n236 = property on="Square" class="Bool (strict)"(error in=w280, "Visible"=w277) -> (error out=w279:errorcluster)  [unwired: 1 in, 1 out]
                n237 = property on="Ampl" class="DigNum (strict)"(error in=w274, "Visible"=w277) -> (error out=w282:errorcluster)  [unwired: 1 in, 1 out]
                n238 = property on="PhaseDBL" class="DigNum (strict)"(error in=w273, "Visible"=w277) -> ()  [unwired: 1 in, 2 out]
                n239 = property on="Ramp" class="Bool (strict)"(error in=w279, "Visible"=w277) -> (error out=w278:errorcluster)  [unwired: 1 in, 1 out]
                n240 = property on="HighL" class="DigNum (strict)"(error in=w282, "Visible"=w277) -> ()  [unwired: 1 in, 2 out]
                n241 = property on="Pulse" class="Bool (strict)"(error in=w278, "Visible"=w277) -> ()  [unwired: 1 in, 2 out]
              }
            }
          }
          frame 4 {
            n242 = case shown="False" w288 {
              tunnel: w289 -> [w292 w311]
              frame True {
                w302 = FALSE ("Visible")
                w298 = FALSE ("Visible")
                n243 = property on="Freq-Period" class="Str"(error in=w292, "Visible"=w302) -> (error out=w308:errorcluster)  [unwired: 1 in, 1 out]
                n244 = property on="Freq/Period" class="Bool (strict)"(error in=w292, "Visible"=w302) -> (error out=w305:errorcluster)  [unwired: 1 in, 1 out]
                n245 = property on="Slider" class="Bool (strict)"("Visible"=TRUE) -> ()  [unwired: 2 in, 2 out]
                n246 = property on="Ampl/HighL" class="Bool (strict)"(error in=w305, "Visible"=w302) -> (error out=w304:errorcluster)  [unwired: 1 in, 1 out]
                n247 = property on="Ampl-HighL" class="Str"(error in=w308, "Visible"=w302) -> (error out=w307:errorcluster)  [unwired: 1 in, 1 out]
                n248 = property on="Offset/LowL" class="Bool (strict)"(error in=w304, "Visible"=w302) -> (error out=w291:errorcluster)  [unwired: 1 in, 1 out]
                n249 = property on="Offset-LowL" class="Str"(error in=w307, "Visible"=w302) -> (error out=w306:errorcluster)  [unwired: 1 in, 1 out]
                n250 = property on="PhaseStr" class="Str"(error in=w306, "Visible"=w302) -> (error out=w297:errorcluster)  [unwired: 1 in, 1 out]
                n251 = property on="Freq" class="DigNum (strict)"(error in=w297, "Visible"=w298) -> (error out=w296:errorcluster)  [unwired: 1 in, 1 out]
                n252 = property on="Offset" class="DigNum (strict)"(error in=w291, "Visible"=w298) -> (error out=w293:errorcluster)  [unwired: 1 in, 1 out]
                n253 = property on="OK" class="Bool (strict)"(error in=w292, "Visible"=w298) -> ()  [unwired: 1 in, 2 out]
                n254 = property on="Sine" class="Bool (strict)"(error in=w292, "Visible"=w298) -> (error out=w301:errorcluster)  [unwired: 1 in, 1 out]
                n255 = property on="Noise" class="Bool (strict)"(error in=w292, "Visible"=w298) -> ()  [unwired: 1 in, 2 out]
                n256 = property on="Period" class="DigNum (strict)"(error in=w296, "Visible"=w298) -> (error out=w295:errorcluster)  [unwired: 1 in, 1 out]
                n257 = property on="LowL" class="DigNum (strict)"(error in=w293, "Visible"=w298) -> (error out=w294:errorcluster)  [unwired: 1 in, 1 out]
                n258 = property on="Square" class="Bool (strict)"(error in=w301, "Visible"=w298) -> (error out=w300:errorcluster)  [unwired: 1 in, 1 out]
                n259 = property on="Ampl" class="DigNum (strict)"(error in=w295, "Visible"=w298) -> (error out=w303:errorcluster)  [unwired: 1 in, 1 out]
                n260 = property on="PhaseDBL" class="DigNum (strict)"(error in=w294, "Visible"=w298) -> ()  [unwired: 1 in, 2 out]
                n261 = property on="Ramp" class="Bool (strict)"(error in=w300, "Visible"=w298) -> (error out=w299:errorcluster)  [unwired: 1 in, 1 out]
                n262 = property on="HighL" class="DigNum (strict)"(error in=w303, "Visible"=w298) -> ()  [unwired: 1 in, 2 out]
                n263 = property on="Pulse" class="Bool (strict)"(error in=w299, "Visible"=w298) -> ()  [unwired: 1 in, 2 out]
              }
              frame False {
                w321 = TRUE ("Visible")
                w317 = FALSE ("Visible")
                n264 = property on="Freq-Period" class="Str"(error in=w311, "Visible"=w321) -> (error out=w327:errorcluster)  [unwired: 1 in, 1 out]
                n265 = property on="Freq/Period" class="Bool (strict)"(error in=w311, "Visible"=w321) -> (error out=w324:errorcluster)  [unwired: 1 in, 1 out]
                n266 = property on="Slider" class="Bool (strict)"("Visible"=TRUE) -> ()  [unwired: 2 in, 2 out]
                n267 = property on="Ampl/HighL" class="Bool (strict)"(error in=w324, "Visible"=w321) -> (error out=w323:errorcluster)  [unwired: 1 in, 1 out]
                n268 = property on="Ampl-HighL" class="Str"(error in=w327, "Visible"=w321) -> (error out=w326:errorcluster)  [unwired: 1 in, 1 out]
                n269 = property on="Offset/LowL" class="Bool (strict)"(error in=w323, "Visible"=w321) -> (error out=w310:errorcluster)  [unwired: 1 in, 1 out]
                n270 = property on="Offset-LowL" class="Str"(error in=w326, "Visible"=w321) -> (error out=w325:errorcluster)  [unwired: 1 in, 1 out]
                n271 = property on="PhaseStr" class="Str"(error in=w325, "Visible"=w321) -> (error out=w316:errorcluster)  [unwired: 1 in, 1 out]
                n272 = property on="Freq" class="DigNum (strict)"(error in=w316, "Visible"=w317) -> (error out=w315:errorcluster)  [unwired: 1 in, 1 out]
                n273 = property on="Offset" class="DigNum (strict)"(error in=w310, "Visible"=w317) -> (error out=w312:errorcluster)  [unwired: 1 in, 1 out]
                n274 = property on="OK" class="Bool (strict)"(error in=w311, "Visible"=w317) -> ()  [unwired: 1 in, 2 out]
                n275 = property on="Sine" class="Bool (strict)"(error in=w311, "Visible"=w317) -> (error out=w320:errorcluster)  [unwired: 1 in, 1 out]
                n276 = property on="Noise" class="Bool (strict)"(error in=w311, "Visible"=w317) -> ()  [unwired: 1 in, 2 out]
                n277 = property on="Period" class="DigNum (strict)"(error in=w315, "Visible"=w317) -> (error out=w314:errorcluster)  [unwired: 1 in, 1 out]
                n278 = property on="LowL" class="DigNum (strict)"(error in=w312, "Visible"=w317) -> (error out=w313:errorcluster)  [unwired: 1 in, 1 out]
                n279 = property on="Square" class="Bool (strict)"(error in=w320, "Visible"=w317) -> (error out=w319:errorcluster)  [unwired: 1 in, 1 out]
                n280 = property on="Ampl" class="DigNum (strict)"(error in=w314, "Visible"=w317) -> (error out=w322:errorcluster)  [unwired: 1 in, 1 out]
                n281 = property on="PhaseDBL" class="DigNum (strict)"(error in=w313, "Visible"=w317) -> ()  [unwired: 1 in, 2 out]
                n282 = property on="Ramp" class="Bool (strict)"(error in=w319, "Visible"=w317) -> (error out=w318:errorcluster)  [unwired: 1 in, 1 out]
                n283 = property on="HighL" class="DigNum (strict)"(error in=w322, "Visible"=w317) -> ()  [unwired: 1 in, 2 out]
                n284 = property on="Pulse" class="Bool (strict)"(error in=w318, "Visible"=w317) -> ()  [unwired: 1 in, 2 out]
              }
            }
          }
          frame 8 {
            n285 = case shown="True" w328 {
              tunnel: w329 -> [w332 w351]
              frame True {
                w342 = FALSE ("Visible")
                w338 = FALSE ("Visible")
                n286 = property on="Freq-Period" class="Str"(error in=w332, "Visible"=w342) -> (error out=w348:errorcluster)  [unwired: 1 in, 1 out]
                n287 = property on="Freq/Period" class="Bool (strict)"(error in=w332, "Visible"=w342) -> (error out=w345:errorcluster)  [unwired: 1 in, 1 out]
                n288 = property on="Slider" class="Bool (strict)"("Visible"=TRUE) -> ()  [unwired: 2 in, 2 out]
                n289 = property on="Ampl/HighL" class="Bool (strict)"(error in=w345, "Visible"=w342) -> (error out=w344:errorcluster)  [unwired: 1 in, 1 out]
                n290 = property on="Ampl-HighL" class="Str"(error in=w348, "Visible"=w342) -> (error out=w347:errorcluster)  [unwired: 1 in, 1 out]
                n291 = property on="Offset/LowL" class="Bool (strict)"(error in=w344, "Visible"=w342) -> (error out=w331:errorcluster)  [unwired: 1 in, 1 out]
                n292 = property on="Offset-LowL" class="Str"(error in=w347, "Visible"=w342) -> (error out=w346:errorcluster)  [unwired: 1 in, 1 out]
                n293 = property on="PhaseStr" class="Str"(error in=w346, "Visible"=w342) -> (error out=w337:errorcluster)  [unwired: 1 in, 1 out]
                n294 = property on="Freq" class="DigNum (strict)"(error in=w337, "Visible"=w338) -> (error out=w336:errorcluster)  [unwired: 1 in, 1 out]
                n295 = property on="Offset" class="DigNum (strict)"(error in=w331, "Visible"=w338) -> (error out=w333:errorcluster)  [unwired: 1 in, 1 out]
                n296 = property on="OK" class="Bool (strict)"(error in=w332, "Visible"=w338) -> ()  [unwired: 1 in, 2 out]
                n297 = property on="Sine" class="Bool (strict)"(error in=w332, "Visible"=w338) -> (error out=w341:errorcluster)  [unwired: 1 in, 1 out]
                n298 = property on="Noise" class="Bool (strict)"(error in=w332, "Visible"=w338) -> ()  [unwired: 1 in, 2 out]
                n299 = property on="Period" class="DigNum (strict)"(error in=w336, "Visible"=w338) -> (error out=w335:errorcluster)  [unwired: 1 in, 1 out]
                n300 = property on="LowL" class="DigNum (strict)"(error in=w333, "Visible"=w338) -> (error out=w334:errorcluster)  [unwired: 1 in, 1 out]
                n301 = property on="Square" class="Bool (strict)"(error in=w341, "Visible"=w338) -> (error out=w340:errorcluster)  [unwired: 1 in, 1 out]
                n302 = property on="Ampl" class="DigNum (strict)"(error in=w335, "Visible"=w338) -> (error out=w343:errorcluster)  [unwired: 1 in, 1 out]
                n303 = property on="PhaseDBL" class="DigNum (strict)"(error in=w334, "Visible"=w338) -> ()  [unwired: 1 in, 2 out]
                n304 = property on="Ramp" class="Bool (strict)"(error in=w340, "Visible"=w338) -> (error out=w339:errorcluster)  [unwired: 1 in, 1 out]
                n305 = property on="HighL" class="DigNum (strict)"(error in=w343, "Visible"=w338) -> ()  [unwired: 1 in, 2 out]
                n306 = property on="Pulse" class="Bool (strict)"(error in=w339, "Visible"=w338) -> ()  [unwired: 1 in, 2 out]
              }
              frame False {
                w361 = TRUE ("Visible")
                w357 = FALSE ("Visible")
                n307 = property on="Freq-Period" class="Str"(error in=w351, "Visible"=w361) -> (error out=w367:errorcluster)  [unwired: 1 in, 1 out]
                n308 = property on="Freq/Period" class="Bool (strict)"(error in=w351, "Visible"=w361) -> (error out=w364:errorcluster)  [unwired: 1 in, 1 out]
                n309 = property on="Slider" class="Bool (strict)"("Visible"=TRUE) -> ()  [unwired: 2 in, 2 out]
                n310 = property on="Ampl/HighL" class="Bool (strict)"(error in=w364, "Visible"=w361) -> (error out=w363:errorcluster)  [unwired: 1 in, 1 out]
                n311 = property on="Ampl-HighL" class="Str"(error in=w367, "Visible"=w361) -> (error out=w366:errorcluster)  [unwired: 1 in, 1 out]
                n312 = property on="Offset/LowL" class="Bool (strict)"(error in=w363, "Visible"=w361) -> (error out=w350:errorcluster)  [unwired: 1 in, 1 out]
                n313 = property on="Offset-LowL" class="Str"(error in=w366, "Visible"=w361) -> (error out=w365:errorcluster)  [unwired: 1 in, 1 out]
                n314 = property on="PhaseStr" class="Str"(error in=w365, "Visible"=w361) -> (error out=w356:errorcluster)  [unwired: 1 in, 1 out]
                n315 = property on="Freq" class="DigNum (strict)"(error in=w356, "Visible"=w357) -> (error out=w355:errorcluster)  [unwired: 1 in, 1 out]
                n316 = property on="Offset" class="DigNum (strict)"(error in=w350, "Visible"=w357) -> (error out=w352:errorcluster)  [unwired: 1 in, 1 out]
                n317 = property on="OK" class="Bool (strict)"(error in=w351, "Visible"=w357) -> ()  [unwired: 1 in, 2 out]
                n318 = property on="Sine" class="Bool (strict)"(error in=w351, "Visible"=w357) -> (error out=w360:errorcluster)  [unwired: 1 in, 1 out]
                n319 = property on="Noise" class="Bool (strict)"(error in=w351, "Visible"=w357) -> ()  [unwired: 1 in, 2 out]
                n320 = property on="Period" class="DigNum (strict)"(error in=w355, "Visible"=w357) -> (error out=w354:errorcluster)  [unwired: 1 in, 1 out]
                n321 = property on="LowL" class="DigNum (strict)"(error in=w352, "Visible"=w357) -> (error out=w353:errorcluster)  [unwired: 1 in, 1 out]
                n322 = property on="Square" class="Bool (strict)"(error in=w360, "Visible"=w357) -> (error out=w359:errorcluster)  [unwired: 1 in, 1 out]
                n323 = property on="Ampl" class="DigNum (strict)"(error in=w354, "Visible"=w357) -> (error out=w362:errorcluster)  [unwired: 1 in, 1 out]
                n324 = property on="PhaseDBL" class="DigNum (strict)"(error in=w353, "Visible"=w357) -> ()  [unwired: 1 in, 2 out]
                n325 = property on="Ramp" class="Bool (strict)"(error in=w359, "Visible"=w357) -> (error out=w358:errorcluster)  [unwired: 1 in, 1 out]
                n326 = property on="HighL" class="DigNum (strict)"(error in=w362, "Visible"=w357) -> ()  [unwired: 1 in, 2 out]
                n327 = property on="Pulse" class="Bool (strict)"(error in=w358, "Visible"=w357) -> ()  [unwired: 1 in, 2 out]
              }
            }
          }
        }
        n328 = case shown="1" w227 {
          tunnel: ["Home_Sine.bmp" w235 w239 w243 "Home_Noise.bmp"] -> w225
          tunnel: w226 -> [_ w234 w238 w242 _]
          frame 1 {
          }
          frame 2, Default {
            n329 = case shown="False" w234 {
              tunnel: ["Home_Square_2.bmp" "Home_Square_1.bmp"] -> w235
              frame True {
              }
              frame False {
              }
            }
          }
          frame 4 {
            n330 = case shown="True" w238 {
              tunnel: ["Home_Ramp_2.bmp" "Home_Ramp_1.bmp"] -> w239
              frame True {
              }
              frame False {
              }
            }
          }
          frame 8 {
            n331 = case shown="False" w242 {
              tunnel: ["Home_Pulse_2.bmp" "Home_Pulse_1.bmp"] -> w243
              frame True {
              }
              frame False {
              }
            }
          }
          frame 16 {
          }
        }
        n332 = Build Path(base path=w230, name or relative path=w225) -> (appended path=w232:path)
        n333 = call "RDG822 Update Screen.vi"("error in"=w228, "Path to file"=w232) -> ("error out"=w229:errorcluster, "Screen"=w231:picture)  [unwired: 8 in]
        n334 = local write "Screen"(w231) -> ()
        n335 = local write "error out"(w229) -> ()
      }
      event "OK": Mouse Down {
        w369 = TRUE ("Visible")
        w368 = FALSE ("Visible")
        # "Добавить слайдер/меню кейсы"
        # "Сделать пересчет"
        n336 = event-data() -> ()  [unwired: 1 in, 8 out]
        n337 = local read "MenuCont"() -> (w380:u32)
        n338 = local read "Slider"() -> (w382:bool)
        n339 = call "Time Delay9"("error in (no error)"=w383) -> ("error out"=w378:errorcluster)  [unwired: 10 in]
        n340 = case shown="1" w380 {
          tunnel: ["Home_Sine.bmp" w410 w417 w424 "Home_Noise.bmp"] -> w381
          tunnel: w382 -> [_ w409 w416 w423 _]
          tunnel: w378 -> [w403 w407 w414 w421 w428]
          tunnel: [w402 w406 w413 w420 w427] -> w377
          frame 1 {
            n341 = property on="Slider" class="Bool (strict)"(error in=w403, "Visible"=FALSE) -> (error out=w402:errorcluster)  [unwired: 1 in, 1 out]
          }
          frame 2, Default {
            n342 = case shown="False" w409 {
              tunnel: ["Home_Square_2.bmp" "Home_Square_1.bmp"] -> w410
              frame True {
              }
              frame False {
              }
            }
            n343 = property on="Slider" class="Bool (strict)"(error in=w407, "Visible"=TRUE) -> (error out=w406:errorcluster)  [unwired: 1 in, 1 out]
          }
          frame 4 {
            n344 = case shown="True" w416 {
              tunnel: ["Home_Ramp_2.bmp" "Home_Ramp_1.bmp"] -> w417
              frame True {
              }
              frame False {
              }
            }
            n345 = property on="Slider" class="Bool (strict)"(error in=w414, "Visible"=TRUE) -> (error out=w413:errorcluster)  [unwired: 1 in, 1 out]
          }
          frame 8 {
            n346 = case shown="False" w423 {
              tunnel: ["Home_Pulse_2.bmp" "Home_Pulse_1.bmp"] -> w424
              frame True {
              }
              frame False {
              }
            }
            n347 = property on="Slider" class="Bool (strict)"(error in=w421, "Visible"=TRUE) -> (error out=w420:errorcluster)  [unwired: 1 in, 1 out]
          }
          frame 16 {
            n348 = property on="Slider" class="Bool (strict)"(error in=w428, "Visible"=FALSE) -> (error out=w427:errorcluster)  [unwired: 1 in, 1 out]
          }
        }
        n349 = Build Path(base path=w387, name or relative path=w381) -> (appended path=w386:path)
        n350 = property on="DutyStr" class="Str"("Visible"=w369) -> ()  [unwired: 2 in, 2 out]
        n351 = call "RDG822 Update Screen.vi"("error in"=w377, "Path to file"=w386) -> ("error out"=w375:errorcluster, "Screen"=w385:picture)  [unwired: 8 in]
        n352 = property on="Freq-Period" class="Str"(error in=w375, "Visible"=w369) -> (error out=w400:errorcluster)  [unwired: 1 in, 1 out]
        n353 = property on="Ampl-HighL" class="Str"(error in=w400, "Visible"=w369) -> (error out=w399:errorcluster)  [unwired: 1 in, 1 out]
        n354 = property on="Offset-LowL" class="Str"(error in=w399, "Visible"=w369) -> (error out=w398:errorcluster)  [unwired: 1 in, 1 out]
        n355 = property on="PhaseStr" class="Str"(error in=w398, "Visible"=w369) -> (error out=w397:errorcluster)  [unwired: 1 in, 1 out]
        n356 = property on="Freq/Period" class="Bool (strict)"(error in=w397, "Visible"=w369) -> (error out=w396:errorcluster)  [unwired: 1 in, 1 out]
        n357 = property on="Ampl/HighL" class="Bool (strict)"(error in=w396, "Visible"=w369) -> (error out=w395:errorcluster)  [unwired: 1 in, 1 out]
        n358 = property on="Offset/LowL" class="Bool (strict)"(error in=w395, "Visible"=w369) -> (error out=w379:errorcluster)  [unwired: 1 in, 1 out]
        n359 = stacked-sequence {
          tunnel: [_ _ w462 _ _] -> w372
          tunnel: [_ w449 _ _ _] -> w373
          tunnel: [w432 _ _ _ _] -> w374
          tunnel: w390 -> [w431 _ _ _ _]
          tunnel: w389 -> [_ w448 _ _ _]
          tunnel: w388 -> [_ _ w461 _ _]
          tunnel: [_ w447 _ _ _] -> w376
          tunnel: w375 -> [_ w447 _ _ _]
          tunnel: [_ _ _ w469 _] -> w371
          tunnel: [_ _ _ _ w492] -> w370
          frame #0 {
            n360 = case shown="False" w431 {
              tunnel: [w434 w441] -> w432
              frame False {
                n361 = local read "Freq"() -> (w437:dbl)
                n362 = Divide(x=1000.0, y=w437) -> (x/y=w436:dbl)
                n363 = Number To Fractional String(number=w437, precision (6)=i16 9) -> (F-format string=w433:string)  [unwired: 2 in]
                n364 = local write "Period"(w436) -> ()
                n365 = Concatenate Strings(w433, " Hz" ("string")) -> (w434:string)
              }
              frame True {
                n366 = local read "Period"() -> (w444:dbl)
                n367 = Divide(x=1000.0, y=w444) -> (x/y=w443:dbl)
                n368 = Number To Fractional String(number=w444, precision (6)=i16 7) -> (F-format string=w440:string)  [unwired: 2 in]
                n369 = local write "Freq"(w443) -> ()
                n370 = Concatenate Strings(w440, " ms" ("string")) -> (w441:string)
              }
            }
          }
          frame #1 {
            n371 = case shown="False" w448 {
              tunnel: [w455 w458] -> w449
              frame False {
                # "Must vary"
                n372 = local read "Ampl"() -> (w454:dbl)
                n373 = In Range and Coerce(upper limit=20.0, x=w454, lower limit=0.002 ("t")) -> (coerced(x)=w451:dbl, In Range?=w450:bool)
                n374 = case shown="False" w450 {
                  frame False {
                    n375 = One Button Dialog(message="Amplitude can`t be less than 2 mA\nor more  than 20 A!") -> ()  [unwired: 1 in, 1 out]
                  }
                  frame True {
                  }
                }
                n376 = Number To Fractional String(number=w451, precision (6)=i16 4) -> (F-format string=w455:string)  [unwired: 2 in]
              }
              frame True {
                n377 = local read "HighL"() -> (w459:dbl)
                n378 = Number To Fractional String(number=w459, precision (6)=i16 4) -> (F-format string=w458:string)  [unwired: 2 in]
              }
            }
          }
          frame #2 {
            n379 = case shown="False" w461 {
              tunnel: [w464 w468] -> w462
              frame False {
                # "Must vary"
                n380 = local read "Offset"() -> (w465:dbl)
                n381 = Number To Fractional String(number=w465, precision (6)=i16 4) -> (F-format string=w464:string)  [unwired: 2 in]
              }
              frame True {
                n382 = local read "LowL"() -> (w466:dbl)
                n383 = Number To Fractional String(number=w466, precision (6)=i16 4) -> (F-format string=w468:string)  [unwired: 2 in]
              }
            }
          }
          frame #3 {
            n384 = local read "PhaseDBL"() -> (w473:dbl)
            n385 = while {
              shift-right: [w475] -> w472
              shift-left: w473 -> [w477]
              stop <- w476 stop-if-true
              w478 = 360.0001 ("upper limit")
              n386 = In Range and Coerce(upper limit=w478, x=w477, lower limit=0.0) -> (In Range?=w476:bool)  [unwired: 1 out]
              n387 = case shown="False" w476 {
                tunnel: w478 -> [w483 _]
                tunnel: w477 -> [w481 w490]
                tunnel: [w480 w490] -> w475
                frame False {
                  n388 = Greater?(x=w481, y=w483) -> (0:w482:bool)
                  n389 = case shown="True" w482 {
                    tunnel: w481 -> [w485 w487]
                    tunnel: [w484 w488] -> w480
                    frame False {
                      n390 = Add(x=w485, y=360.0) -> (x+y=w484:dbl)
                    }
                    frame True {
                      n391 = Subtract(x=w487, y=360.0) -> (x-y=w488:dbl)
                    }
                  }
                }
                frame True {
                }
              }
            }
            n392 = Number To Fractional String(number=w472, precision (6)=i16 3) -> (F-format string=w470:string)  [unwired: 2 in]
            n393 = Concatenate Strings(w470, " °" ("string")) -> (w469:string)
          }
          frame #4 {
            n394 = local read "DutyDBL"() -> (w495:dbl)
            n395 = while {
              shift-right: [w497] -> w494
              shift-left: w495 -> [w499]
              stop <- w498 stop-if-true
              w500 = 100.0001 ("upper limit")
              n396 = In Range and Coerce(upper limit=w500, x=w499, lower limit=0.0) -> (In Range?=w498:bool)  [unwired: 1 out]
              n397 = case shown="False" w498 {
                tunnel: w500 -> [w505 _]
                tunnel: w499 -> [w503 w512]
                tunnel: [w502 w512] -> w497
                frame False {
                  n398 = Greater?(x=w503, y=w505) -> (0:w504:bool)
                  n399 = case shown="False" w504 {
                    tunnel: w503 -> [w507 w509]
                    tunnel: [w506 w510] -> w502
                    frame False {
                      n400 = Add(x=w507, y=100.0) -> (x+y=w506:dbl)
                    }
                    frame True {
                      n401 = Subtract(x=w509, y=100.0) -> (x-y=w510:dbl)
                    }
                  }
                }
                frame True {
                }
              }
            }
            n402 = Number To Fractional String(number=w494, precision (6)=i16 3) -> (F-format string=w491:string)  [unwired: 2 in]
            n403 = Concatenate Strings(w491, " %" ("string")) -> (w492:string)
          }
        }
        n404 = property on="Offset" class="DigNum (strict)"("Visible"=w368) -> (error out=w391:errorcluster)  [unwired: 2 in, 1 out]
        n405 = property on="PhaseDBL" class="DigNum (strict)"("Visible"=w368) -> ()  [unwired: 2 in, 2 out]
        n406 = property on="Freq" class="DigNum (strict)"(error in=w379, "Visible"=w368) -> (error out=w394:errorcluster)  [unwired: 1 in, 1 out]
        n407 = property on="OK" class="Bool (strict)"("Visible"=w368) -> (error out=w384:errorcluster)  [unwired: 2 in, 1 out]
        n408 = property on="LowL" class="DigNum (strict)"(error in=w391, "Visible"=w368) -> ()  [unwired: 1 in, 2 out]
        n409 = property on="DutyDBL" class="DigNum (strict)"("Visible"=w368) -> ()  [unwired: 2 in, 2 out]
        n410 = property on="Period" class="DigNum (strict)"(error in=w394, "Visible"=w368) -> (error out=w393:errorcluster)  [unwired: 1 in, 1 out]
        n411 = property on="Ampl" class="DigNum (strict)"(error in=w393, "Visible"=w368) -> (error out=w392:errorcluster)  [unwired: 1 in, 1 out]
        n412 = property on="HighL" class="DigNum (strict)"(error in=w392, "Visible"=w368) -> ()  [unwired: 1 in, 2 out]
        n413 = call "Time Delay3"("error in (no error)"=w384) -> ("error out"=w401:errorcluster)  [unwired: 10 in]
        n414 = property on="OK" class="Bool (strict)"(error in=w401, "Value"=w368) -> ()  [unwired: 1 in, 2 out]
        n415 = local write "Freq-Period"(w374) -> ()
        n416 = local write "Ampl-HighL"(w373) -> ()
        n417 = local write "Offset-LowL"(w372) -> ()
        n418 = local write "PhaseStr"(w371) -> ()
        n419 = local write "DutyStr"(w370) -> ()
        n420 = local write "error out"(w376) -> ()
        n421 = local write "Screen"(w385) -> ()
      }
      event "Freq-Period": Mouse Down {
        w514 = FALSE ("Visible")
        n422 = event-data() -> ()  [unwired: 1 in, 8 out]
        n423 = property on="Freq-Period" class="Str"("Visible"=w514) -> (error out=w532:errorcluster)  [unwired: 2 in, 1 out]
        n424 = property on="Ampl-HighL" class="Str"(error in=w532, "Visible"=w514) -> (error out=w528:errorcluster)  [unwired: 1 in, 1 out]
        n425 = property on="Offset-LowL" class="Str"(error in=w528, "Visible"=w514) -> (error out=w524:errorcluster)  [unwired: 1 in, 1 out]
        n426 = property on="PhaseStr" class="Str"(error in=w524, "Visible"=w514) -> (error out=w523:errorcluster)  [unwired: 1 in, 1 out]
        n427 = property on="Freq/Period" class="Bool (strict)"(error in=w523, "Visible"=w514) -> (error out=w531:errorcluster)  [unwired: 1 in, 1 out]
        n428 = property on="Ampl/HighL" class="Bool (strict)"(error in=w531, "Visible"=w514) -> (error out=w527:errorcluster)  [unwired: 1 in, 1 out]
        n429 = property on="Offset/LowL" class="Bool (strict)"(error in=w527, "Visible"=w514) -> (error out=w515:errorcluster)  [unwired: 1 in, 1 out]
        n430 = property on="Slider" class="Bool (strict)"(error in=w515, "Visible"=w514) -> (error out=w513:errorcluster)  [unwired: 1 in, 1 out]
        n431 = property on="Freq" class="DigNum (strict)"(error in=w513, "Visible"=w514) -> (error out=w534:errorcluster)  [unwired: 1 in, 1 out]
        n432 = property on="Period" class="DigNum (strict)"(error in=w534, "Visible"=w514) -> (error out=w530:errorcluster)  [unwired: 1 in, 1 out]
        n433 = property on="Ampl" class="DigNum (strict)"(error in=w530, "Visible"=w514) -> (error out=w529:errorcluster)  [unwired: 1 in, 1 out]
        n434 = property on="HighL" class="DigNum (strict)"(error in=w529, "Visible"=w514) -> (error out=w526:errorcluster)  [unwired: 1 in, 1 out]
        n435 = property on="Offset" class="DigNum (strict)"(error in=w526, "Visible"=w514) -> (error out=w525:errorcluster)  [unwired: 1 in, 1 out]
        n436 = property on="LowL" class="DigNum (strict)"(error in=w525, "Visible"=w514) -> (error out=w521:errorcluster)  [unwired: 1 in, 1 out]
        n437 = property on="PhaseDBL" class="DigNum (strict)"(error in=w521, "Visible"=w514) -> (error out=w517:errorcluster)  [unwired: 1 in, 1 out]
        n438 = case shown="False" w533 {
          tunnel: [w541 w547] -> w520
          tunnel: w535 -> [w539 w545]
          tunnel: w517 -> [w537 w543]
          tunnel: [w536 w542] -> w519
          frame False {
            n439 = property on="Freq" class="DigNum (strict)"(error in=w537, "Visible"=TRUE) -> (error out=w536:errorcluster)  [unwired: 1 in, 1 out]
            n440 = Build Path(base path=w539, name or relative path="Freq.bmp") -> (appended path=w541:path)
          }
          frame True {
            n441 = property on="Period" class="DigNum (strict)"(error in=w543, "Visible"=TRUE) -> (error out=w542:errorcluster)  [unwired: 1 in, 1 out]
            n442 = Build Path(base path=w545, name or relative path="Period.bmp") -> (appended path=w547:path)
          }
        }
        n443 = call "RDG822 Update Screen.vi"("error in"=w519, "Path to file"=w520) -> ("error out"=w518:errorcluster, "Screen"=w516:picture)  [unwired: 8 in]
        n444 = local write "Screen"(w516) -> ()
        n445 = property on="OK" class="Bool (strict)"("Visible"=TRUE) -> ()  [unwired: 2 in, 2 out]
      }
      event "Ampl-HighL": Mouse Down {
        w550 = FALSE ("Visible")
        n446 = event-data() -> ()  [unwired: 1 in, 8 out]
        n447 = property on="Freq-Period" class="Str"("Visible"=w550) -> (error out=w568:errorcluster)  [unwired: 2 in, 1 out]
        n448 = property on="Ampl-HighL" class="Str"(error in=w568, "Visible"=w550) -> (error out=w563:errorcluster)  [unwired: 1 in, 1 out]
        n449 = property on="Offset-LowL" class="Str"(error in=w563, "Visible"=w550) -> (error out=w559:errorcluster)  [unwired: 1 in, 1 out]
        n450 = property on="PhaseStr" class="Str"(error in=w559, "Visible"=w550) -> (error out=w558:errorcluster)  [unwired: 1 in, 1 out]
        n451 = property on="Freq/Period" class="Bool (strict)"(error in=w558, "Visible"=w550) -> (error out=w567:errorcluster)  [unwired: 1 in, 1 out]
        n452 = property on="Ampl/HighL" class="Bool (strict)"(error in=w567, "Visible"=w550) -> (error out=w562:errorcluster)  [unwired: 1 in, 1 out]
        n453 = property on="Offset/LowL" class="Bool (strict)"(error in=w562, "Visible"=w550) -> (error out=w549:errorcluster)  [unwired: 1 in, 1 out]
        n454 = property on="Slider" class="Bool (strict)"(error in=w549, "Visible"=w550) -> (error out=w548:errorcluster)  [unwired: 1 in, 1 out]
        n455 = property on="Freq" class="DigNum (strict)"(error in=w548, "Visible"=w550) -> (error out=w569:errorcluster)  [unwired: 1 in, 1 out]
        n456 = property on="Period" class="DigNum (strict)"(error in=w569, "Visible"=w550) -> (error out=w566:errorcluster)  [unwired: 1 in, 1 out]
        n457 = property on="Ampl" class="DigNum (strict)"(error in=w566, "Visible"=w550) -> (error out=w564:errorcluster)  [unwired: 1 in, 1 out]
        n458 = property on="HighL" class="DigNum (strict)"(error in=w564, "Visible"=w550) -> (error out=w561:errorcluster)  [unwired: 1 in, 1 out]
        n459 = property on="Offset" class="DigNum (strict)"(error in=w561, "Visible"=w550) -> (error out=w560:errorcluster)  [unwired: 1 in, 1 out]
        n460 = property on="LowL" class="DigNum (strict)"(error in=w560, "Visible"=w550) -> (error out=w556:errorcluster)  [unwired: 1 in, 1 out]
        n461 = property on="PhaseDBL" class="DigNum (strict)"(error in=w556, "Visible"=w550) -> (error out=w555:errorcluster)  [unwired: 1 in, 1 out]
        n462 = case shown="True" w565 {
          tunnel: [w576 w582] -> w554
          tunnel: w570 -> [w574 w580]
          tunnel: w555 -> [w572 w579]
          tunnel: [w571 w577] -> w553
          frame False {
            n463 = property on="Ampl" class="DigNum (strict)"(error in=w572, "Visible"=TRUE) -> (error out=w571:errorcluster)  [unwired: 1 in, 1 out]
            n464 = Build Path(base path=w574, name or relative path="Ampl.bmp") -> (appended path=w576:path)
          }
          frame True {
            n465 = property on="HighL" class="DigNum (strict)"(error in=w579, "Visible"=TRUE) -> (error out=w577:errorcluster)  [unwired: 1 in, 1 out]
            n466 = Build Path(base path=w580, name or relative path="HighL.bmp") -> (appended path=w582:path)
          }
        }
        n467 = call "RDG822 Update Screen.vi"("error in"=w553, "Path to file"=w554) -> ("error out"=w552:errorcluster, "Screen"=w551:picture)  [unwired: 8 in]
        n468 = local write "Screen"(w551) -> ()
        n469 = property on="OK" class="Bool (strict)"("Visible"=TRUE) -> ()  [unwired: 2 in, 2 out]
      }
      event "Offset-LowL": Mouse Down {
        w585 = FALSE ("Visible")
        n470 = event-data() -> ()  [unwired: 1 in, 8 out]
        n471 = property on="Freq-Period" class="Str"("Visible"=w585) -> (error out=w603:errorcluster)  [unwired: 2 in, 1 out]
        n472 = property on="Ampl-HighL" class="Str"(error in=w603, "Visible"=w585) -> (error out=w599:errorcluster)  [unwired: 1 in, 1 out]
        n473 = property on="Offset-LowL" class="Str"(error in=w599, "Visible"=w585) -> (error out=w595:errorcluster)  [unwired: 1 in, 1 out]
        n474 = property on="PhaseStr" class="Str"(error in=w595, "Visible"=w585) -> (error out=w594:errorcluster)  [unwired: 1 in, 1 out]
        n475 = property on="Freq/Period" class="Bool (strict)"(error in=w594, "Visible"=w585) -> (error out=w602:errorcluster)  [unwired: 1 in, 1 out]
        n476 = property on="Ampl/HighL" class="Bool (strict)"(error in=w602, "Visible"=w585) -> (error out=w598:errorcluster)  [unwired: 1 in, 1 out]
        n477 = property on="Offset/LowL" class="Bool (strict)"(error in=w598, "Visible"=w585) -> (error out=w584:errorcluster)  [unwired: 1 in, 1 out]
        n478 = property on="Slider" class="Bool (strict)"(error in=w584, "Visible"=w585) -> (error out=w583:errorcluster)  [unwired: 1 in, 1 out]
        n479 = property on="Freq" class="DigNum (strict)"(error in=w583, "Visible"=w585) -> (error out=w604:errorcluster)  [unwired: 1 in, 1 out]
        n480 = property on="Period" class="DigNum (strict)"(error in=w604, "Visible"=w585) -> (error out=w601:errorcluster)  [unwired: 1 in, 1 out]
        n481 = property on="Ampl" class="DigNum (strict)"(error in=w601, "Visible"=w585) -> (error out=w600:errorcluster)  [unwired: 1 in, 1 out]
        n482 = property on="HighL" class="DigNum (strict)"(error in=w600, "Visible"=w585) -> (error out=w596:errorcluster)  [unwired: 1 in, 1 out]
        n483 = property on="Offset" class="DigNum (strict)"(error in=w596, "Visible"=w585) -> (error out=w597:errorcluster)  [unwired: 1 in, 1 out]
        n484 = property on="LowL" class="DigNum (strict)"(error in=w597, "Visible"=w585) -> (error out=w591:errorcluster)  [unwired: 1 in, 1 out]
        n485 = property on="PhaseDBL" class="DigNum (strict)"(error in=w591, "Visible"=w585) -> (error out=w590:errorcluster)  [unwired: 1 in, 1 out]
        n486 = case shown="False" w593 {
          tunnel: [w611 w617] -> w589
          tunnel: w605 -> [w609 w615]
          tunnel: w590 -> [w607 w614]
          tunnel: [w606 w612] -> w588
          frame False {
            n487 = property on="Offset" class="DigNum (strict)"(error in=w607, "Visible"=TRUE) -> (error out=w606:errorcluster)  [unwired: 1 in, 1 out]
            n488 = Build Path(base path=w609, name or relative path="Offset.bmp") -> (appended path=w611:path)
          }
          frame True {
            n489 = property on="LowL" class="DigNum (strict)"(error in=w614, "Visible"=TRUE) -> (error out=w612:errorcluster)  [unwired: 1 in, 1 out]
            n490 = Build Path(base path=w615, name or relative path="LowL.bmp") -> (appended path=w617:path)
          }
        }
        n491 = call "RDG822 Update Screen.vi"("error in"=w588, "Path to file"=w589) -> ("error out"=w587:errorcluster, "Screen"=w586:picture)  [unwired: 8 in]
        n492 = local write "Screen"(w586) -> ()
        n493 = property on="OK" class="Bool (strict)"("Visible"=TRUE) -> ()  [unwired: 2 in, 2 out]
      }
      event "PhaseStr": Mouse Down {
        w620 = FALSE ("Visible")
        n494 = event-data() -> ()  [unwired: 1 in, 8 out]
        n495 = property on="Freq-Period" class="Str"("Visible"=w620) -> (error out=w640:errorcluster)  [unwired: 2 in, 1 out]
        n496 = property on="Ampl-HighL" class="Str"(error in=w640, "Visible"=w620) -> (error out=w636:errorcluster)  [unwired: 1 in, 1 out]
        n497 = property on="Offset-LowL" class="Str"(error in=w636, "Visible"=w620) -> (error out=w632:errorcluster)  [unwired: 1 in, 1 out]
        n498 = property on="PhaseStr" class="Str"(error in=w632, "Visible"=w620) -> (error out=w631:errorcluster)  [unwired: 1 in, 1 out]
        n499 = property on="Freq/Period" class="Bool (strict)"(error in=w631, "Visible"=w620) -> (error out=w639:errorcluster)  [unwired: 1 in, 1 out]
        n500 = property on="Ampl/HighL" class="Bool (strict)"(error in=w639, "Visible"=w620) -> (error out=w635:errorcluster)  [unwired: 1 in, 1 out]
        n501 = property on="Offset/LowL" class="Bool (strict)"(error in=w635, "Visible"=w620) -> (error out=w619:errorcluster)  [unwired: 1 in, 1 out]
        n502 = property on="Slider" class="Bool (strict)"(error in=w619, "Visible"=w620) -> (error out=w618:errorcluster)  [unwired: 1 in, 1 out]
        n503 = property on="Freq" class="DigNum (strict)"(error in=w618, "Visible"=w620) -> (error out=w641:errorcluster)  [unwired: 1 in, 1 out]
        n504 = property on="Period" class="DigNum (strict)"(error in=w641, "Visible"=w620) -> (error out=w638:errorcluster)  [unwired: 1 in, 1 out]
        n505 = property on="Ampl" class="DigNum (strict)"(error in=w638, "Visible"=w620) -> (error out=w637:errorcluster)  [unwired: 1 in, 1 out]
        n506 = property on="HighL" class="DigNum (strict)"(error in=w637, "Visible"=w620) -> (error out=w633:errorcluster)  [unwired: 1 in, 1 out]
        n507 = property on="Offset" class="DigNum (strict)"(error in=w633, "Visible"=w620) -> (error out=w634:errorcluster)  [unwired: 1 in, 1 out]
        n508 = property on="LowL" class="DigNum (strict)"(error in=w634, "Visible"=w620) -> (error out=w627:errorcluster)  [unwired: 1 in, 1 out]
        n509 = property on="PhaseDBL" class="DigNum (strict)"(error in=w627, "Visible"=w620) -> (error out=w626:errorcluster)  [unwired: 1 in, 1 out]
        n510 = property on="PhaseDBL" class="DigNum (strict)"(error in=w626, "Visible"=TRUE) -> (error out=w623:errorcluster)  [unwired: 1 in, 1 out]
        n511 = Build Path(base path=w629, name or relative path="Phase.bmp") -> (appended path=w624:path)
        n512 = call "RDG822 Update Screen.vi"("error in"=w623, "Path to file"=w624) -> ("error out"=w622:errorcluster, "Screen"=w621:picture)  [unwired: 8 in]
        n513 = local write "Screen"(w621) -> ()
        n514 = property on="OK" class="Bool (strict)"("Visible"=TRUE) -> ()  [unwired: 2 in, 2 out]
      }
      event "DutyStr": Mouse Down {
        w642 = FALSE ("Visible")
        n515 = event-data() -> ()  [unwired: 1 in, 8 out]
        n516 = property on="Freq-Period" class="Str"("Visible"=w642) -> (error out=w661:errorcluster)  [unwired: 2 in, 1 out]
        n517 = property on="Freq/Period" class="Bool (strict)"("Visible"=w642) -> (error out=w660:errorcluster)  [unwired: 2 in, 1 out]
        n518 = property on="Freq" class="DigNum (strict)"("Visible"=w642) -> (error out=w662:errorcluster)  [unwired: 2 in, 1 out]
        n519 = property on="Offset" class="DigNum (strict)"("Visible"=w642) -> (error out=w655:errorcluster)  [unwired: 2 in, 1 out]
        n520 = property on="Ampl-HighL" class="Str"(error in=w661, "Visible"=w642) -> (error out=w657:errorcluster)  [unwired: 1 in, 1 out]
        n521 = property on="Ampl/HighL" class="Bool (strict)"(error in=w660, "Visible"=w642) -> (error out=w656:errorcluster)  [unwired: 1 in, 1 out]
        n522 = property on="Period" class="DigNum (strict)"(error in=w662, "Visible"=w642) -> (error out=w659:errorcluster)  [unwired: 1 in, 1 out]
        n523 = property on="LowL" class="DigNum (strict)"(error in=w655, "Visible"=w642) -> (error out=w650:errorcluster)  [unwired: 1 in, 1 out]
        n524 = property on="Offset-LowL" class="Str"(error in=w657, "Visible"=w642) -> (error out=w654:errorcluster)  [unwired: 1 in, 1 out]
        n525 = property on="Offset/LowL" class="Bool (strict)"(error in=w656, "Visible"=w642) -> (error out=w643:errorcluster)  [unwired: 1 in, 1 out]
        n526 = property on="Ampl" class="DigNum (strict)"(error in=w659, "Visible"=w642) -> (error out=w658:errorcluster)  [unwired: 1 in, 1 out]
        n527 = property on="PhaseDBL" class="DigNum (strict)"(error in=w650, "Visible"=w642) -> (error out=w649:errorcluster)  [unwired: 1 in, 1 out]
        n528 = property on="DutyDBL" class="DigNum (strict)"(error in=w649, "Visible"=TRUE) -> (error out=w646:errorcluster)  [unwired: 1 in, 1 out]
        n529 = property on="PhaseStr" class="Str"(error in=w654, "Visible"=w642) -> ()  [unwired: 1 in, 2 out]
        n530 = property on="Slider" class="Bool (strict)"(error in=w643, "Visible"=w642) -> ()  [unwired: 1 in, 2 out]
        n531 = property on="HighL" class="DigNum (strict)"(error in=w658, "Visible"=w642) -> ()  [unwired: 1 in, 2 out]
        n532 = property on="DutyDBL" class="DigNum (strict)"("Visible"=w642) -> ()  [unwired: 2 in, 2 out]
        n533 = Build Path(base path=w652, name or relative path="Duty.bmp") -> (appended path=w647:path)
        n534 = property on="DutyStr" class="Str"("Visible"=w642) -> ()  [unwired: 2 in, 2 out]
        n535 = call "RDG822 Update Screen.vi"("error in"=w646, "Path to file"=w647) -> ("error out"=w645:errorcluster, "Screen"=w644:picture)  [unwired: 8 in]
        n536 = local write "Screen"(w644) -> ()
        n537 = property on="OK" class="Bool (strict)"("Visible"=TRUE) -> ()  [unwired: 2 in, 2 out]
      }
      event "Freq/Period": Value Change {
        n538 = event-data() -> ("NewVal"=w663:bool)  [unwired: 1 in, 5 out]
        n539 = case shown="False" w663 {
          tunnel: [w667 w673] -> w664
          frame False {
            # "Must vary"
            n540 = local read "Period"() -> (w670:dbl)
            n541 = Divide(x=1000.0, y=w670) -> (x/y=w668:dbl)
            n542 = Number To Fractional String(number=w668, precision (6)=i16 9) -> (F-format string=w665:string)  [unwired: 2 in]
            n543 = local write "Freq"(w668) -> ()
            n544 = Concatenate Strings(w665, " Hz" ("string")) -> (w667:string)
          }
          frame True {
            # "Must vary"
            n545 = local read "Freq"() -> (w676:dbl)
            n546 = Divide(x=1000.0, y=w676) -> (x/y=w675:dbl)
            n547 = local write "Period"(w675) -> ()
            n548 = Number To Fractional String(number=w675, precision (6)=i16 7) -> (F-format string=w672:string)  [unwired: 2 in]
            n549 = Concatenate Strings(w672, " ms" ("string")) -> (w673:string)
          }
        }
        n550 = local write "Freq-Period"(w664) -> ()
      }
      event "Ampl/HighL", "Offset/LowL": Value Change {
        # "Переделать"
        # "Сделать пересчет"
        n551 = event-data() -> ("NewVal"=w681:bool)  [unwired: 1 in, 5 out]
        n552 = case shown="False" w681 {
          tunnel: [w685 w689] -> w682
          frame False {
            # "Must vary"
            n553 = local read "Offset"() -> (w686:dbl)
            n554 = Number To Fractional String(number=w686, precision (6)=i16 4) -> (F-format string=w685:string)  [unwired: 2 in]
          }
          frame True {
            n555 = local read "LowL"() -> (w687:dbl)
            n556 = Number To Fractional String(number=w687, precision (6)=i16 4) -> (F-format string=w689:string)  [unwired: 2 in]
          }
        }
        n557 = case shown="False" w681 {
          tunnel: [w691 w695] -> w683
          frame False {
            # "Must vary"
            n558 = local read "Ampl"() -> (w692:dbl)
            n559 = Number To Fractional String(number=w692, precision (6)=i16 4) -> (F-format string=w691:string)  [unwired: 2 in]
          }
          frame True {
            n560 = local read "HighL"() -> (w693:dbl)
            n561 = Number To Fractional String(number=w693, precision (6)=i16 4) -> (F-format string=w695:string)  [unwired: 2 in]
          }
        }
        n562 = local read "Ampl/HighL"() -> (w680:bool)
        n563 = local read "Offset/LowL"() -> (w679:bool)
        n564 = local write "Ampl-HighL"(w683) -> ()
        n565 = local write "Offset-LowL"(w682) -> ()
        n566 = local write "Offset/LowL"(w680) -> ()
        n567 = local write "Ampl/HighL"(w679) -> ()
      }
      event "Out1": Mouse Down {
        w703 = 0 items=["Vpp", "Vrms", "dBm"] ("Amplitude Unit (0: Vpp)")
        w717 = u16 2 items=["Send", "Read", "Download", "Remove"] ("Send/Read/Download/Remove")
        w718 = u16 0 items=["Send", "Read", "Download", "Remove"] ("Send/Read/Download/Remove")
        w706 = FALSE ("Visible")
        w721 = 1 items=["Channel 1"=1, "Channel 2"=2] ("Output Channel (1: Channel 1)")
        n568 = event-data() -> ()  [unwired: 1 in, 8 out]
        n569 = case shown="False" w740 {
          tunnel: w739 -> [w799 _]
          tunnel: w738 -> [_ w801]
          tunnel: [w799 w800] -> w701
          frame False {
            # "Freq"
          }
          frame True {
            # "Period"
            n570 = Divide(x=1000.0, y=w801) -> (x/y=w800:dbl)
          }
        }
        n571 = case shown="False" w741 {
          tunnel: w737 -> [w785 _]
          tunnel: w734 -> [_ w797]
          tunnel: [w786 w791] -> w698
          tunnel: w735 -> [_ w796]
          frame False {
            # "Ampl"
            n572 = In Range and Coerce(upper limit=20.0, x=w785, lower limit=0.002 ("t")) -> (coerced(x)=w786:dbl, In Range?=w787:bool)
            n573 = case shown="False" w787 {
              frame False {
                n574 = One Button Dialog(message="Amplitude can`t be less than 2 mA\nor more than 20 A!") -> ()  [unwired: 1 in, 1 out]
              }
              frame True {
              }
            }
          }
          frame True {
            # "High-Low"
            n575 = Subtract(x=w797, y=w796) -> (x-y=w793:dbl)
            n576 = In Range and Coerce(upper limit=20.0, x=w793, lower limit=0.002 ("t")) -> (coerced(x)=w791:dbl, In Range?=w792:bool)
            n577 = case shown="False" w792 {
              frame False {
                n578 = One Button Dialog(message="Amplitude can`t be less than 2 mA\nor greater than 20 A!") -> ()  [unwired: 1 in, 1 out]
              }
              frame True {
              }
            }
          }
        }
        n579 = case shown="True" w736 {
          tunnel: w700 -> [w779 _]
          tunnel: w735 -> [_ w784]
          tunnel: [w779 w780] -> w699
          tunnel: w734 -> [_ w781]
          frame False {
            # "Offset"
          }
          frame True {
            # "HOffset"
            n580 = Add(x=w781, y=w784) -> (x+y=w783:dbl)
            n581 = Divide(x=w783, y=2.0) -> (x/y=w780:dbl)
          }
        }
        n582 = while {
          shift-right: [w763] -> w702
          shift-left: w728 -> [w765]
          stop <- w764 stop-if-true
          w766 = 360.0001 ("upper limit")
          # "Phase"
          n583 = In Range and Coerce(upper limit=w766, x=w765, lower limit=0.0) -> (In Range?=w764:bool)  [unwired: 1 out]
          n584 = case shown="False" w764 {
            tunnel: w766 -> [w771 _]
            tunnel: w765 -> [w769 w778]
            tunnel: [w768 w778] -> w763
            frame False {
              n585 = Greater?(x=w769, y=w771) -> (0:w770:bool)
              n586 = case shown="True" w770 {
                tunnel: w769 -> [w773 w775]
                tunnel: [w772 w776] -> w768
                frame False {
                  n587 = Add(x=w773, y=360.0) -> (x+y=w772:dbl)
                }
                frame True {
                  n588 = Subtract(x=w775, y=360.0) -> (x-y=w776:dbl)
                }
              }
            }
            frame True {
            }
          }
        }
        n589 = while {
          shift-right: [w742] -> w696
          shift-left: w697 -> [w744]
          stop <- w743 stop-if-true
          w745 = 100.0001 ("upper limit")
          # "Duty"
          n590 = In Range and Coerce(upper limit=w745, x=w744, lower limit=0.0) -> (In Range?=w743:bool)  [unwired: 1 out]
          n591 = case shown="False" w743 {
            tunnel: w743 -> [_ _]
            tunnel: w745 -> [w749 w757]
            tunnel: [w748 w757] -> w742
            tunnel: w744 -> [w747 _]
            frame False {
              n592 = Greater?(x=w749, y=w747) -> (0:w750:bool)
              n593 = case shown="False" w750 {
                tunnel: w749 -> [w752 w754]
                tunnel: [w751 w755] -> w748
                frame False {
                  n594 = Add(x=w752, y=100.0) -> (x+y=w751:dbl)
                }
                frame True {
                  n595 = Subtract(x=w754, y=100.0) -> (x-y=w755:dbl)
                }
              }
            }
            frame True {
            }
          }
        }
        n596 = call "RDG822 Standard Waveform.vi"("Amplitude (0.1 Vpp)"=w698, "Frequency (1000 Hz)"=w701, "DC Offset (0.00 V)"=w699, "Output Channel (1: Channel 1)"=w721, "Amplitude Unit (0: Vpp)"=w703, "Phase (0 Degree)"=w702, "error in (no error)"=w723, "Duty Cycle (50 %)"=w696) -> ("resulting string"=w704:string, "error out"=w720:errorcluster)  [unwired: 6 in]
        n597 = call "HTTPGetRequest_Inst.vi"("Send/Read/Download/Remove"=w718, "error in (no error)"=w720, "userdata="=w704, "userID"=w722) -> ("error out"=w710:errorcluster, "ReqNum"=w708:string)  [unwired: 5 in, 1 out]
        n598 = Build Path(base path=w711, name or relative path=path "Results") -> (appended path=w713:path)
        n599 = call "QueryDoneFlag.vi"("error in (no error)"=w710, "ReqNum"=w708) -> ("error out"=w709:errorcluster)  [unwired: 9 in]
        n600 = call "HTTPGetRequest_Inst.vi"("Send/Read/Download/Remove"=w717, "Path to FP"=w713, "error in (no error)"=w709, "ReqNum"=w708) -> ("error out"=w724:errorcluster)  [unwired: 5 in, 2 out]
        n601 = call "UnZipFile.vi"("error in (no error)"=w724, "Zip name"=w708, "Path to FP"=w713) -> ("error out"=w719:errorcluster, "File path"=w715:path)  [unwired: 7 in]
        n602 = case shown="True" "RemoveReq?" {
          tunnel: w719 -> [w758 w762]
          tunnel: [w758 w761] -> w705
          tunnel: w708 -> [_ w759]
          frame False {
          }
          frame True {
            w760 = u16 3 items=["Send", "Read", "Download", "Remove"] ("Send/Read/Download/Remove")
            n603 = call "HTTPGetRequest_Inst.vi"("Send/Read/Download/Remove"=w760, "error in (no error)"=w762, "ReqNum"=w759) -> ("error out"=w761:errorcluster)  [unwired: 6 in, 2 out]
          }
        }
        n604 = property on="Freq-Period" class="Str"(error in=w705, "Visible"=w706) -> (error out=w731:errorcluster)  [unwired: 1 in, 1 out]
        n605 = property on="Freq/Period" class="Bool (strict)"(error in=w705, "Visible"=w706) -> (error out=w727:errorcluster)  [unwired: 1 in, 1 out]
        n606 = property on="Ampl/HighL" class="Bool (strict)"(error in=w727, "Visible"=w706) -> (error out=w726:errorcluster)  [unwired: 1 in, 1 out]
        n607 = property on="Ampl-HighL" class="Str"(error in=w731, "Visible"=w706) -> (error out=w730:errorcluster)  [unwired: 1 in, 1 out]
        n608 = call "Time Delay5"() -> ("error out"=w733:errorcluster)  [unwired: 11 in]
        n609 = call "RDG822 Update Screen.vi"("error in"=w705, "Path to file"=w715) -> ("error out"=w725:errorcluster, "Screen"=w716:picture)  [unwired: 8 in]
        n610 = property on="Offset/LowL" class="Bool (strict)"(error in=w726, "Visible"=w706) -> (error out=w707:errorcluster)  [unwired: 1 in, 1 out]
        n611 = property on="Offset-LowL" class="Str"(error in=w730, "Visible"=w706) -> (error out=w729:errorcluster)  [unwired: 1 in, 1 out]
        n612 = local write "error out"(w725) -> ()
        n613 = property on="Out1" class="Bool (strict)"(error in=w733, "Value"=FALSE ("Out1")) -> ()  [unwired: 1 in, 2 out]
        n614 = local write "Screen"(w716) -> ()
        n615 = property on="Slider" class="Bool (strict)"(error in=w707, "Visible"=w706) -> ()  [unwired: 1 in, 2 out]
        n616 = property on="PhaseStr" class="Str"(error in=w729, "Visible"=w706) -> ()  [unwired: 1 in, 2 out]
      }
      event "Out2": Value Change {
        (unwired) 2 items=["Channel 1"=1, "Channel 2"=2] ("Output Channel (1: Channel 1)")
        # "Same as Out1 eventually"
        n617 = event-data() -> ()  [unwired: 1 in, 6 out]
      }
    }
  }
